vi "Module - Page Setup.vi"(11 "Stop":bool) -> ()   [LabVIEW 2020]
uses:
  Control/Setup - Sequence Data.ctl
  Control/Setup - Sequence Data Label.ctl
  Control/Setup - State.ctl
  Control/Data to Execute.ctl
  Control/Transaction Info.ctl
  Control/Product Info.ctl
  Control/Acceptance Criteria Info.ctl
  Control/Execution Info.ctl
  Control/Results Info.ctl
  Control/State - FGV.ctl
  Control/State - eFGV.ctl
  Control/Section.ctl
  <vilib>/Utility/NIReport.llb/Report Type.ctl
  7311f70c-db24-4098-937e-a840d3f1464f.vi
  babc2730-5d00-47f3-8067-32ba08f41054.vi
  b5994df8-9a62-4c2b-b0b7-1cda760cb50f.vi
  133289ce-597c-4077-9071-527faaeab83e.vi
  50162af0-f45e-4f35-a68f-88f28c3fa732.vi
  <vilib>/Utility/config.llb/Read Key (String).vi
  <vilib>/addons/_office/excel.llb/Excel Get Data ([str]).vi
  <vilib>/Comparison/Equal/Equal Functor/Equal Functor.lvclass
  <vilib>/Utility/NIReport.llb/NI_report.lvclass
  <vilib>/Utility/config.llb/NI_LVConfig.lvlib
  <vilib>/Utility/file.llb/Read Delimited Spreadsheet (string).vi
  <vilib>/Utility/NIReport.llb/NI_ReportGenerationCore.lvlib
  <vilib>/Utility/NIReport.llb/Excel/NI_Excel.lvclass
  <vilib>/addons/_office/NI_ReportGenerationToolkit.lvlib
panel:
  in  "Load Excel":bool
  in  "template (empty)":path
  in  "Tab Control":enum32{"Tests", "Misc."}(tab)=enum."Misc."
  in  "Btn.ClearRunSequence":bool caption="Run All"
  in  "Btn.RunSequence":bool caption="Run All"
  in  "ComboBox.SelectTestSequence":string(combo) caption="Test Sequence"
  in  "Remove Multi test":bool caption="Remove Sensor"
  in  "Add Multi test":bool caption="Add Sensor"
  in  "Header multi-test 3":T1={"Seq.SelectRun 4"="Select", "Seq.Done"="Status", "Seq.No"="Run?", "Seq.No 2"="Test Sequence", "Seq.No 3"="No.", "Seq.No 4"="Test Req. ID", "Seq.No 5"="Test Requirement", "Seq.No 6"="Variance", "Seq.No 7"="Test Procedure", "Seq.No 8"="Section", "Seq.No 9"="Test Bunker", "Seq.No 10"="Test Media", "Seq.No 11"="Test Pressure (psi)", "Seq.No 12"="Cycle", "Seq.No 13"="Holding time (hh:mm)", "Seq.No 14"="Chart Scale", "Seq.No 15"="Blowdown? (y/n)", "Seq.No 16"="Actuator Pressure (psi)", "Seq.No 17"="Max. Blowdown Pressure (psi)"}
  in  "MCListbox.Sequence List":T2[](array[typedef])
  in  "Enum.Permitted Hold Pressure Drop":enum16{"%", "psi"}(ring)
  in  "Enum.Max Start Hold Pressure":enum16{"%", "psi"}(ring)
  in  "Add Additional Ref Procedure":bool caption="Add Sensor"
  in  "Remove Additional Ref Procedure":bool caption="Remove Sensor"
  in  "Remove Sensor":bool
  in  "Add Tool":bool caption="Add Sensor"
  in  "Remove Tools":bool caption="Remove Sensor"
  in  "Add Sensor":bool
  in  "List.Tool":string(combo)
  in  "Header.Tool":T3={"Type "="Type", "Id"=" ID", "Description"="Description", "Serial No"="Serial No"} caption="Header Tool"
  in  "Label.Tools":string="Tools" caption="Tools"
  out "Output Set Description":string caption="Output Set Company"
  in  "ListBox.Output Set":string(combo)="1001.xltx" caption="Output Set"
  in  "Label.Result":string="Result" caption="Result"
  in  "List.Sensor":string(combo)
  in  "Label.Sensor":string="Sensor" caption="Sensor"
  out "Indicator.Sub Operation":string caption="Sub Operation"
  out "Indicator.Confirmation No":u32 caption="Confirmation No"
  out "Indicator.Operation":string caption="Operation"
  out "Indicator.Sequence No":u16 caption="Sequence No"
  in  "Label.Production Order Details":string="Production Order Details" caption="Production Order Details"
  out "Indicator.Order Number":u32 caption="Order Number"
  in  "Table.Procedure No./Ref.":i32(listbox)
  in  "Label.Execution":string="Execution" caption="Execution"
  in  "Label.Acceptance Criteria":string="Acceptance Criteria" caption="Acceptance Criteria"
  in  "Auto Stop Test":bool caption="Automatic Stop Test after Hold Time Countdown"
  in  "Auto Set Marker":bool=TRUE caption="Automatic set start marker upon pressure stabilized"
  in  "Permitted Hold Pressure Drop":dbl=3.0 caption="Permitted Holding Pressure Drop" min=0.0 max=100.0
  in  "Max Start Hold Pressure":dbl=3.0 caption="Maximum Start Of Holding Pressure" min=0.0 max=100.0
  in  "Listbox.PSL":string(combo) caption="PSL"
  in  "Listbox.Rev.":string(combo) caption="Rev."
  in  "Listbox.Additional Procedures No./Ref.":string(combo) caption="Additional Procedures No./Ref."
  in  "Label.Additional Procedures No./Ref.":string="Additional Procedures No./Ref." caption="Additional Procedures No./Ref."
  in  "Table.Sensor":i32(listbox) caption="Detail Sensor"
  in  "Header.Sensor":T4={"Type "="Type", "Id"=" ID", "Description"="Description", "Serial No"="Serial No", "LP"="LP"} caption="Header Detail Sensor"
  in  "Table.Tool":i32(listbox) caption="Detail Sensor"
  in  "Pressure Unit":string
  in  "List SN":i32(listbox)
  in  "Test System Description":string
  in  "Rework":bool caption="Rework?"
  in  "Ref Order No.":dbl caption="Ref. Order No."
  in  "NCR No.":string
  in  "Sales Order":u32
  in  "Procedure No./Ref.":string(combo) caption="Test Document No./Ref."
  in  "Save":bool
  in  "Edit":bool
  in  "Tab Control 2":T5(tab)
  in  "New":bool
  in  "Copy":bool
  in  "Remove SN":bool
  in  "Add SN":bool
  in  "Auto":bool
  in  "Notes":string
  in  "Input SN":string
  out "Working Pressure":string
  in  "Test Category":string
  in  "Test System":string(combo)
  in  "PSL":string
  in  "Rev.":string
  in  "Product Category":string(combo)
  in  "BOM Rev.":dbl
  in  "Material Description":string
  in  "Material":u32
  in  "Item No.":u32
  in  "Project":string
  in  "Customer Description":string
  in  "Customer":u32
  in  "Quantity":u16=1 min=1 step=1
  in  "Order Number":u32
  in  "Search":bool
  in  "Transaction Number":u32 caption="Transaction No."
  # "SETUP"
  # "PSL"
  # "Rev."
  # "on top of the test pressure"
  # "per hour (vs. start holding pressure)"
  # "Maximum Start of Holding Pressure"
  # "Pressure Holding Pressure Drop"
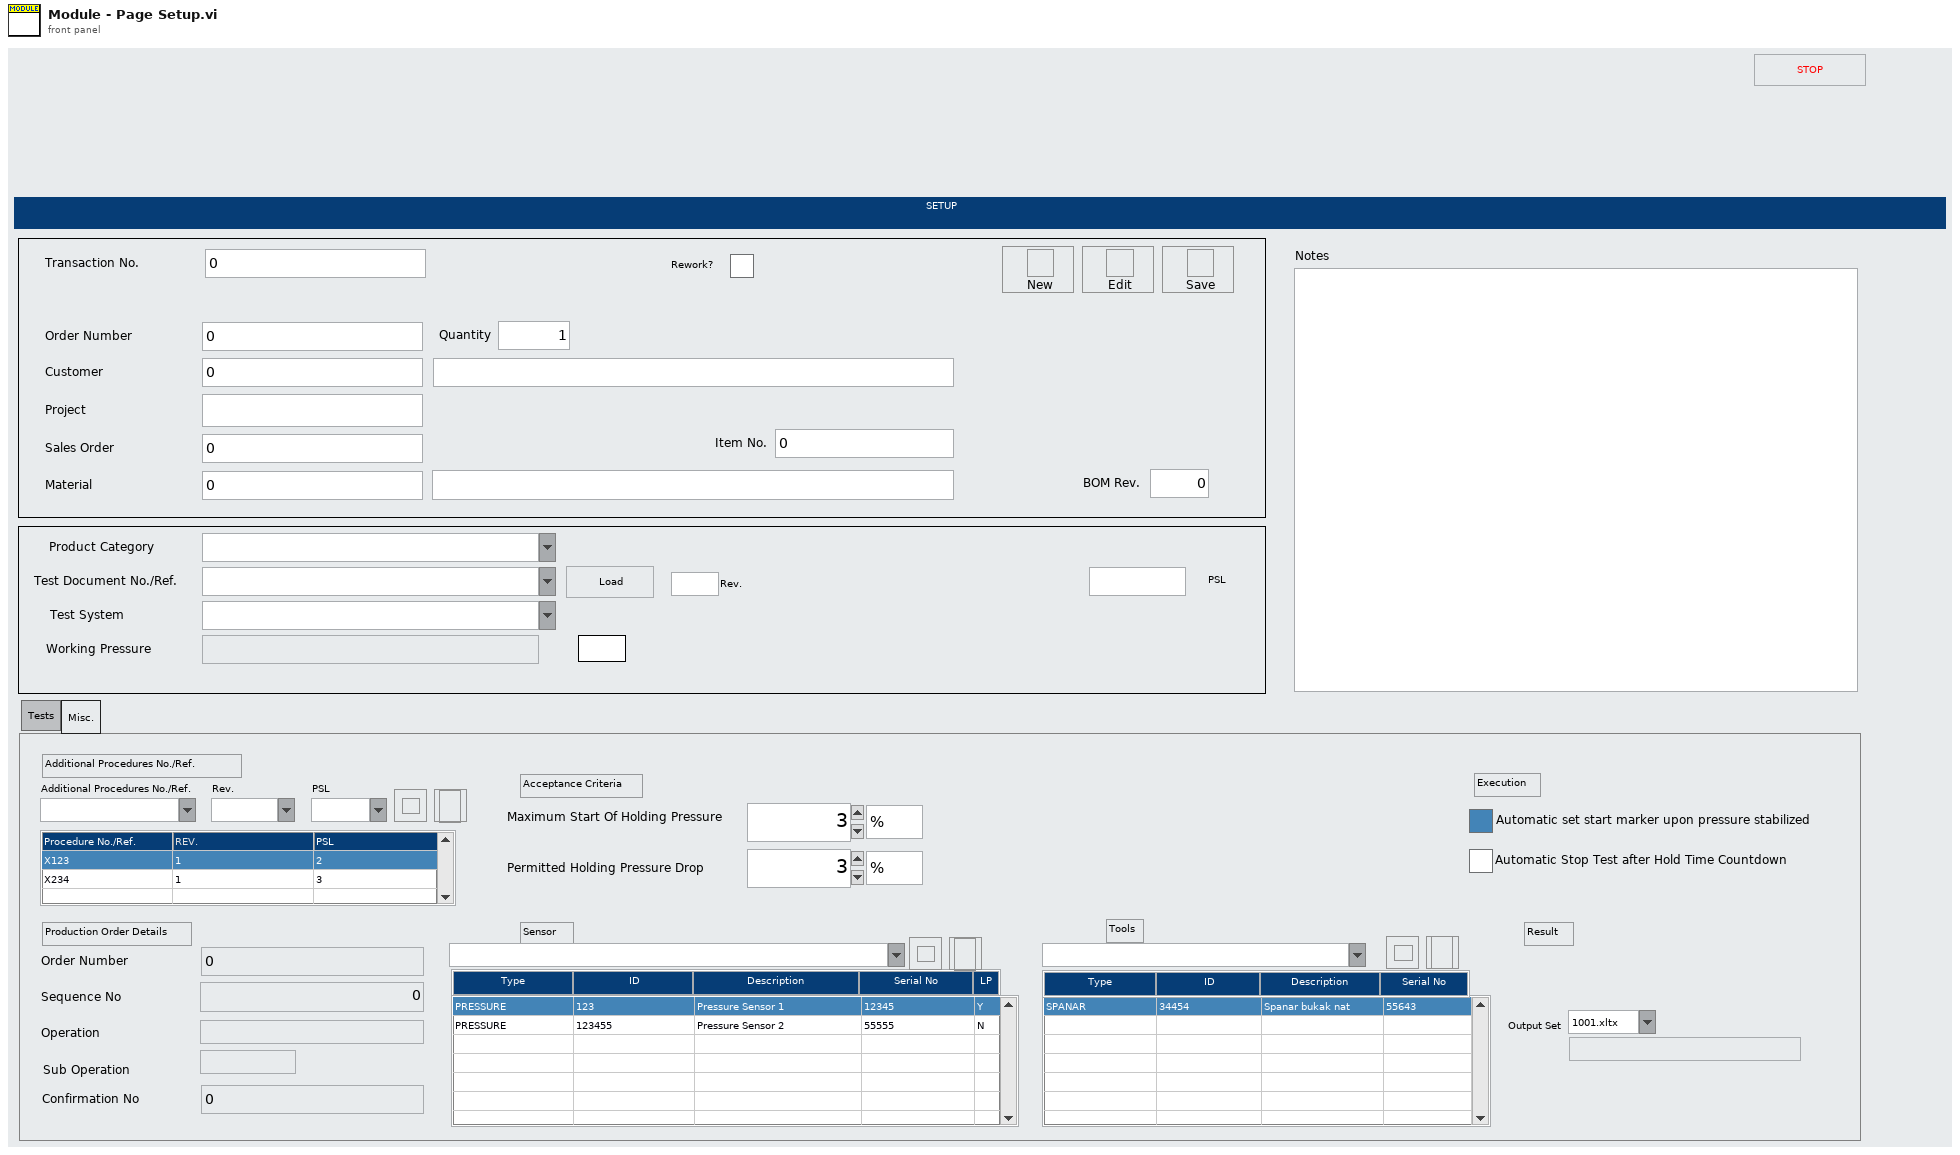
[diagram p1: front panel]
types:
  T1 = typedef "Setup - Sequence Data Label.ctl" = cluster{"Seq.SelectRun 4":string, "Seq.Done":string, "Seq.No":string, "Seq.No 2":string, "Seq.No 3":string, "Seq.No 4":string, "Seq.No 5":string, "Seq.No 6":string, "Seq.No 7":string, "Seq.No 8":string, "Seq.No 9":string, "Seq.No 10":string, "Seq.No 11":string, "Seq.No 12":string, "Seq.No 13":string, "Seq.No 14":string, "Seq.No 15":string, "Seq.No 16":string, "Seq.No 17":string}
  T2 = typedef "Setup - Sequence Data.ctl" = cluster{"Seq.Select":bool, "Seq.Status":u32, "Seq.Run":bool, "Seq.TestSequence":string, "Seq.No":string, "Seq.ReqID":string, "Seq.TestReq":string, "Seq.Variance":string, "Seq.TestProcedure":string, "Seq.Section":string, "Seq.TestBunker":string, "Seq.TestMedia":string, "Seq.TestPressure":string, "Seq.Cycle":string, "Seq.HoldingTime":string, "Seq.ChartScale":string, "Seq.BDIndicator":string, "Seq.ActuatorPressure":string, "Seq.MaxBDPressure":string}
  T3 = cluster{"Type ":string, "Id":string, "Description":string, "Serial No":string}
  T4 = cluster{"Type ":string, "Id":string, "Description":string, "Serial No":string, "LP":string}
  T5 = enum32{"Others                ", "Multi-tests       "}
  T6 = typedef "Data to Execute.ctl" = cluster{"Transaction Info":T7, "Product Info":T8, "Misc - Additional Refs":string[][], "Misc - Sensors":string[][], "Misc - Tools":string[][], "Acceptance Criteria Info":T9, "Execution Info":T10, "Results Info":T11, "Notes":string}
  T7 = typedef "Transaction Info.ctl" = cluster{"Transaction Number":u32, "Order Number":u32, "Quantity":u16, "Customer":u32, "Customer Description":string, "Project":string, "Sales Order":u32, "Material":u32, "Material Description":string, "Rework":bool, "NCR No.":string, "Ref Order No.":dbl, "Item No.":u32, "BOM Rev.":dbl}
  T8 = typedef "Product Info.ctl" = cluster{"Product Category":string, "Procedure No./Ref.":string, "Test System":string, "Test System Description":string, "Working Pressure":string, "Pressure Unit":string, "Rev.":string, "PSL":string}
  T9 = typedef "Acceptance Criteria Info.ctl" = cluster{"Max Start Hold Pressure":dbl, "Enum.Max Start Hold Pressure":enum16{"%", "psi"}, "Permitted Hold Pressure Drop":dbl, "Enum.Permitted Hold Pressure Drop":enum16{"%", "psi"}}
  T10 = typedef "Execution Info.ctl" = cluster{"Auto Set Marker":bool, "Auto Stop Test":bool}
  T11 = typedef "Results Info.ctl" = cluster{"ListBox.Output Set":string, "Output Set Description":string}
  T12 = cluster{"T_Out":i32, "Event Ref":refnum<event-registration>, "Product Category":string, "Seq.AllList":T2[], "Seq.ShownList":T2[], "Seq.HiddenList":T2[], "Procedure No.":string, "File String":string[], "Data to Execute":T6}
  T13 = typedef "Setup - State.ctl" = enum16{"Init", "Register Event", "Read Config File", "Get Output Set List", "Idle", "Get product info", "Read sequence csv", "Get Sequence List", "Get Transaction Info", "Get product Info", "Get Misc - Additional Refs", "Get Misc - Sensors", "Get Misc - Tools", "Get Misc - Accept Criteria", "Get Misc - Execution", "Get Misc - Results", "Get Misc - Notes", "Check Folder Exist", "Create Folder", "Send to Execute", "Close"}
  T14 = typedef "State - FGV.ctl" = enum16{"Write", "Read"}
  T15 = typedef "State - eFGV.ctl" = enum16{"Init", "Read", "Write", "Exit"}
  T16 = typedef "Section.ctl" = enum16{"Software Setup", "Config", "Setup", "Network Stream", "MQTT Client", "Setting", "Sample Interval", "Calibration", "Pre-Ranging", "Overrun", "Static", "Filter", "Properties", "Alarm", "Device", "Logging"}
  T17 = enum8{"Enabled", "Disabled", "Disabled and Grayed Out"}
  T18 = enum16{"maximized", "minimized", "normal", "no change"}
  T19 = typedef "NI_ReportGenerationCore.lvlib/Report Type.ctl" = enum16{"HTML", "Word", "Excel"}
  T20 = typedef "NI_LVConfig.lvlib/Config Data RefNum.ctl" = refnum<k1>
  T21 = cluster{"Type":string, "ID":string, "Description":string, "Serial No.":string, "Low Pressure?":bool}
  T22 = cluster{"Type":string, "ID":string, "Description":string, "Serial No.":string}
  T23 = cluster{"Transaction Number":u32, "Order Number":u32, "Quantity":u16, "Customer":u32, "Customer Description":string, "Project":string, "Sales Order":u32, "Material":u32, "Material Description":string, "Rework":bool, "NCR No.":string, "Ref Order No.":dbl, "Item No.":u32, "BOM Rev.":dbl}
  T24 = cluster{"Product Category":string, "Procedure No./Ref.":string, "Test System":string, "Test System Description":string, "Working Pressure":string, "Pressure Unit":string, "Rev.":string, "PSL":string}
  T25 = cluster{"Max Start Hold Pressure":dbl, "Enum.Max Start Hold Pressure":enum16{"%", "psi"}, "Permitted Hold Pressure Drop":dbl, "Enum.Permitted Hold Pressure Drop":enum16{"%", "psi"}}
  T26 = cluster{"Auto Set Marker":bool, "Auto Stop Test":bool}
  T27 = cluster{"ListBox.Output Set":string, "Output Set Description":string}
  T28 = enum32{"invalid app kind", "Development System", "Run Time System", "Student Edition", "Embedded LabVIEW", "Evaluation", "Custom"}
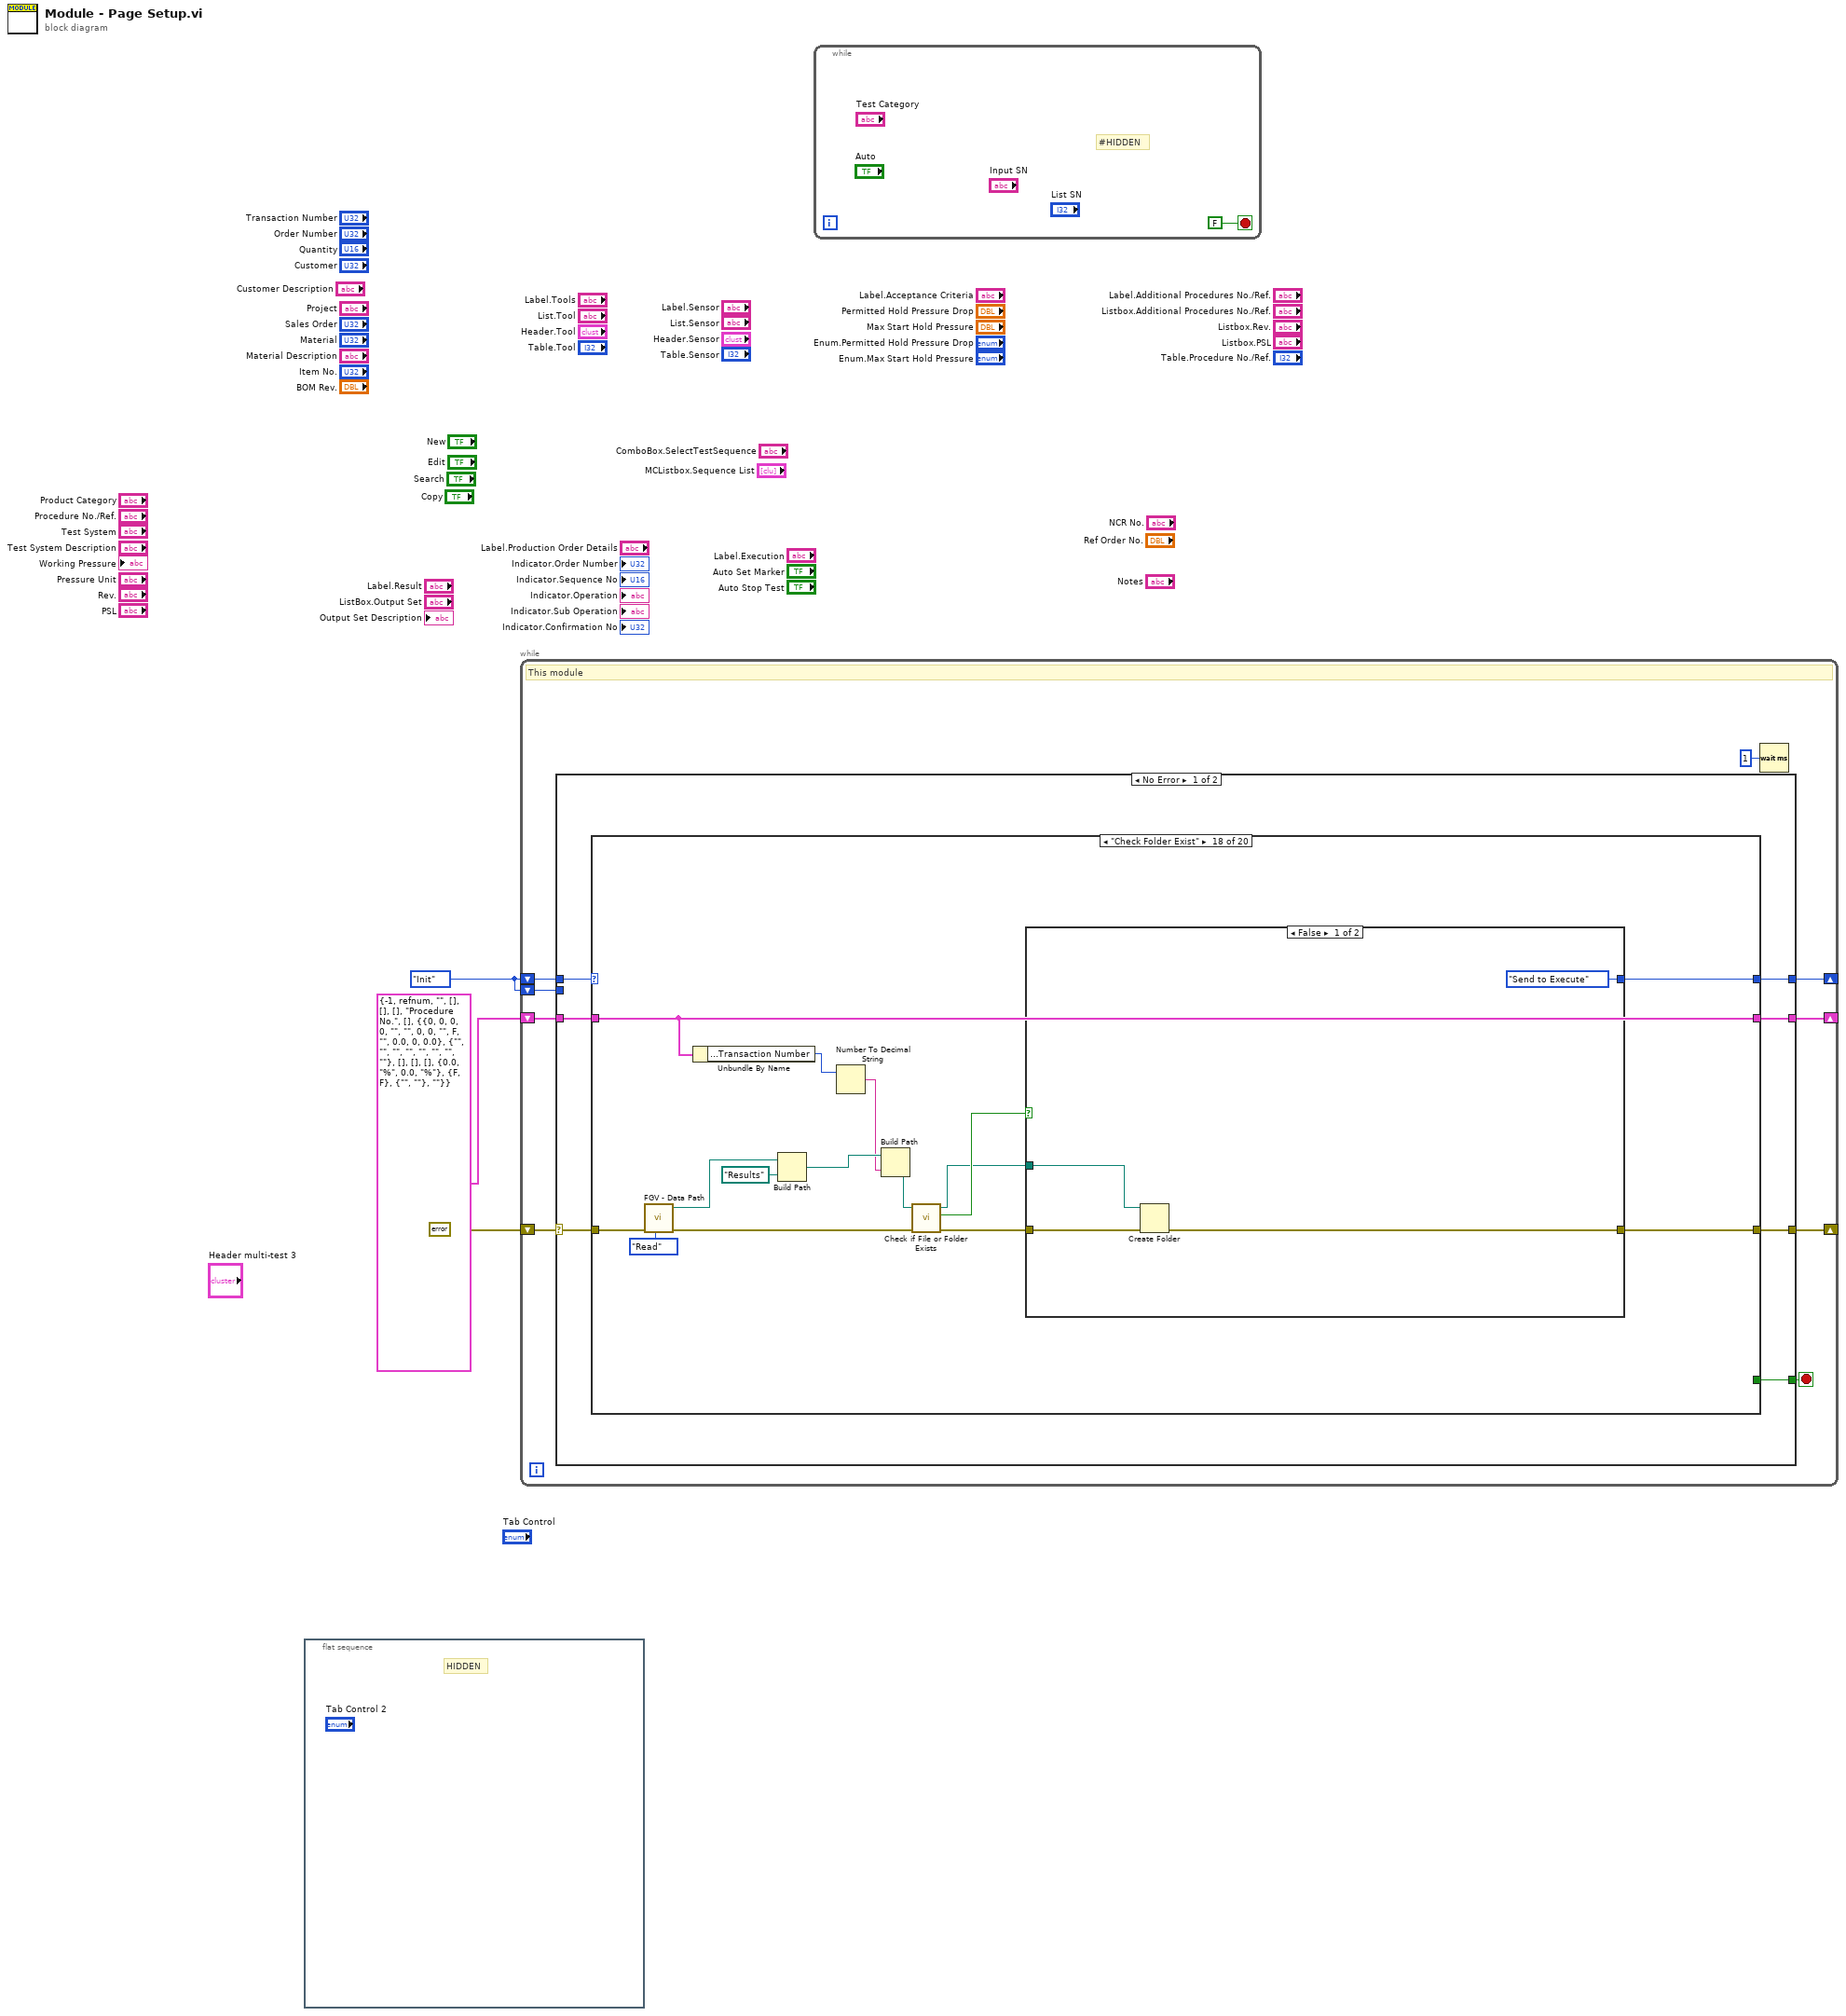
[diagram p0: block diagram]
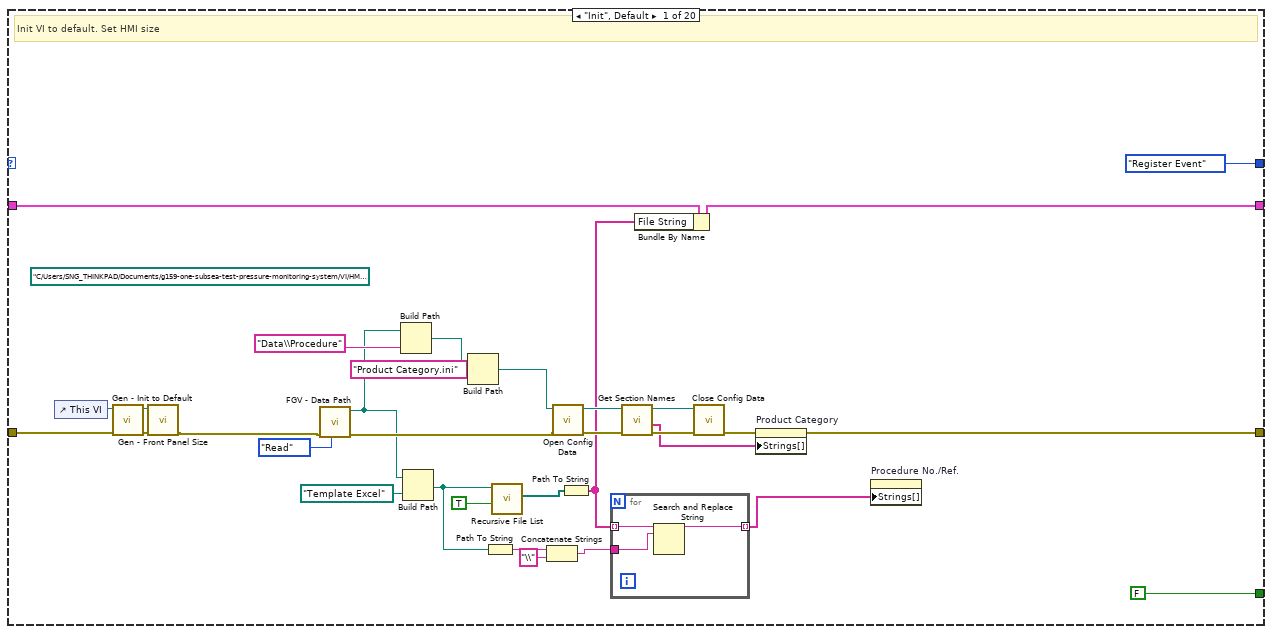
[diagram p2: hidden frame]
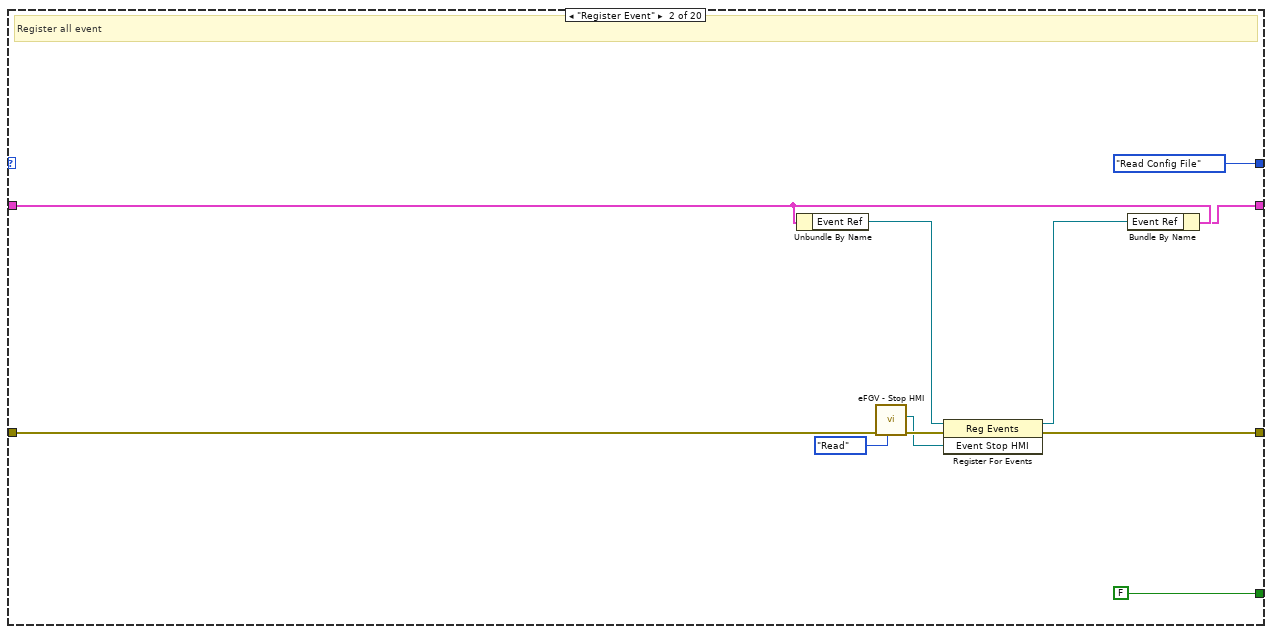
[diagram p3: hidden frame]
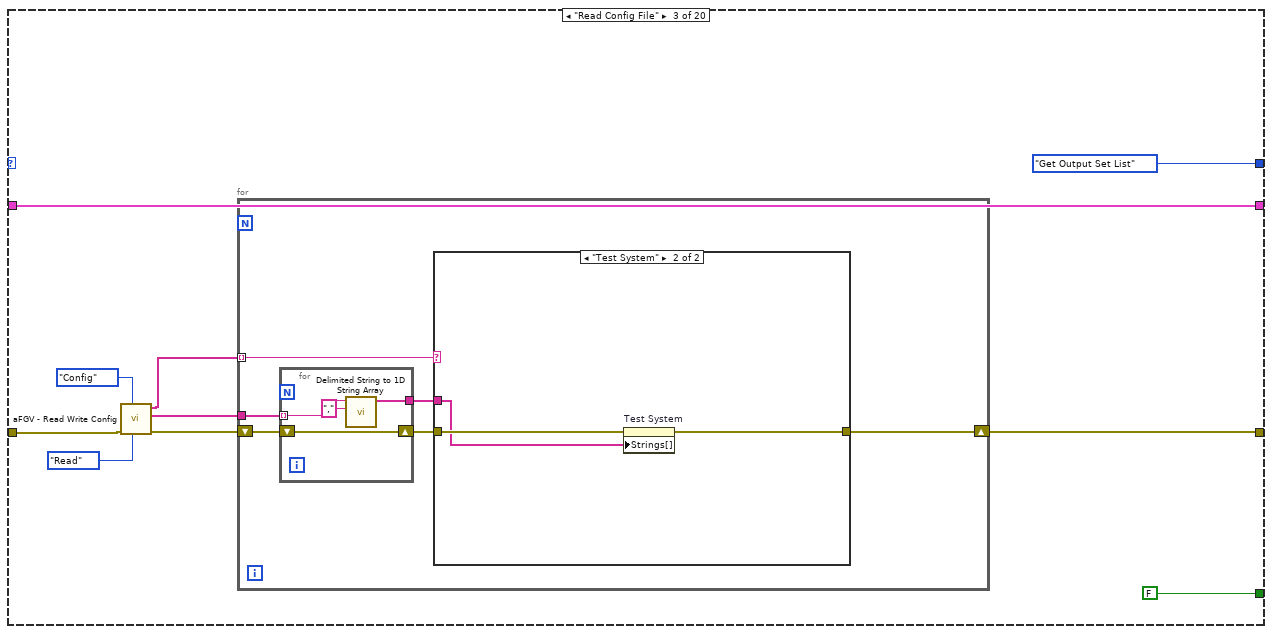
[diagram p4: hidden frame]
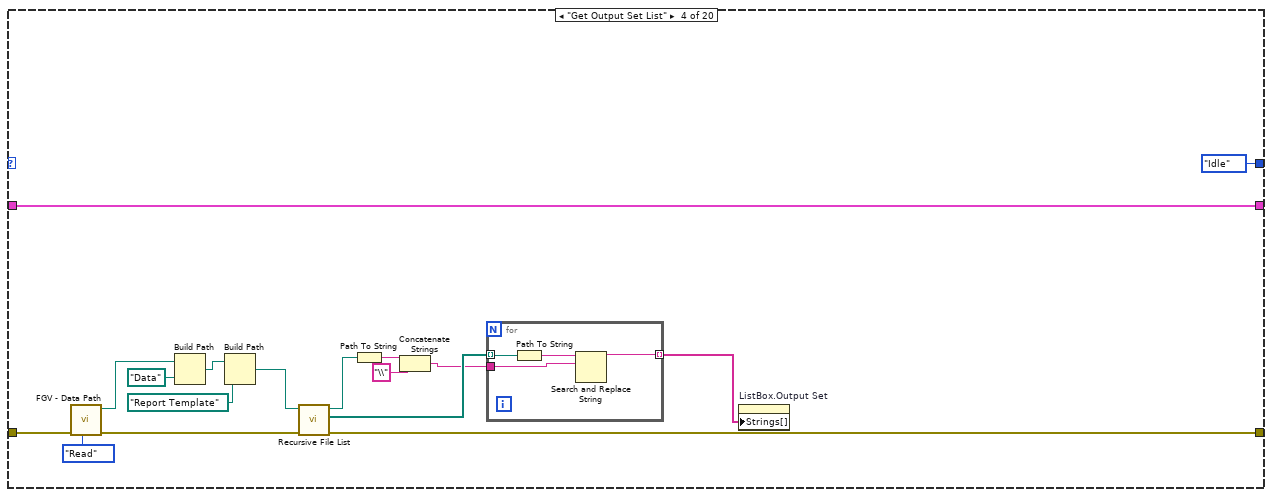
[diagram p6: hidden frame]
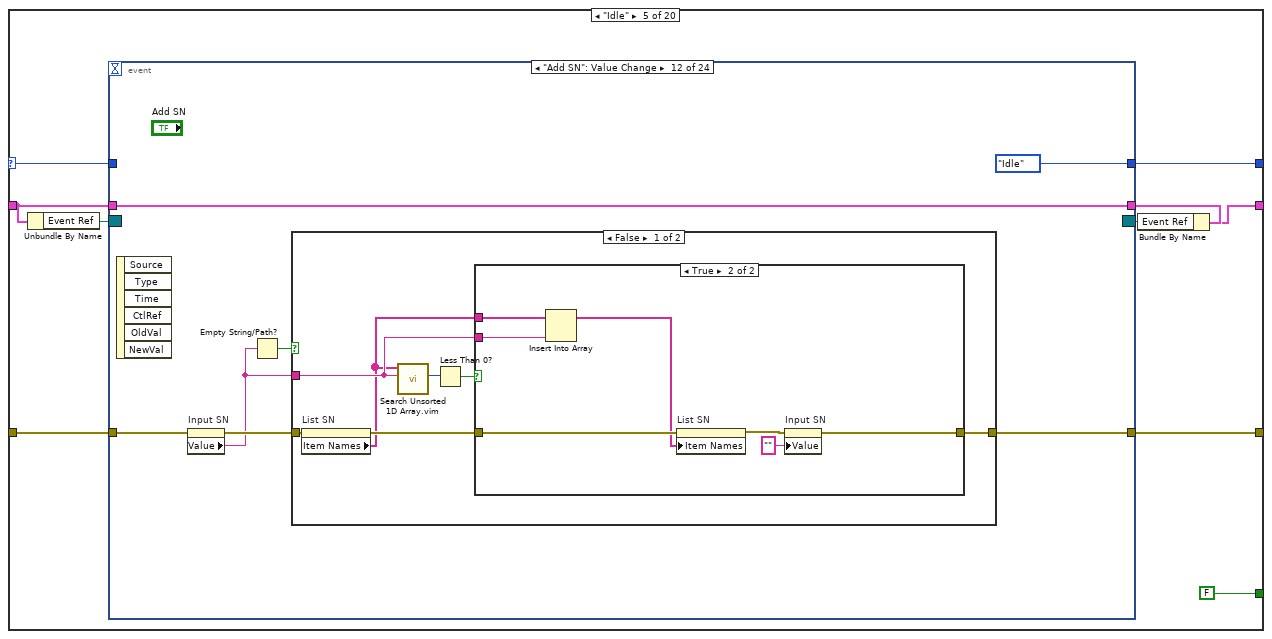
[diagram p7: hidden frame]
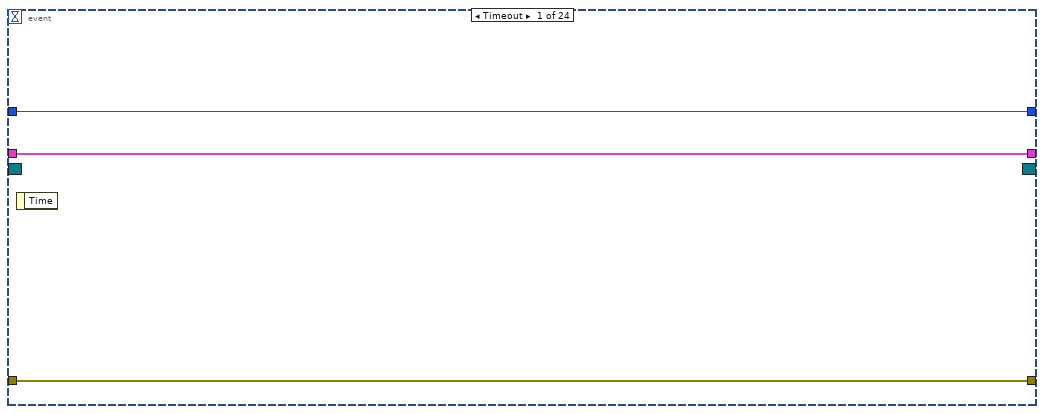
[diagram p8: hidden frame]
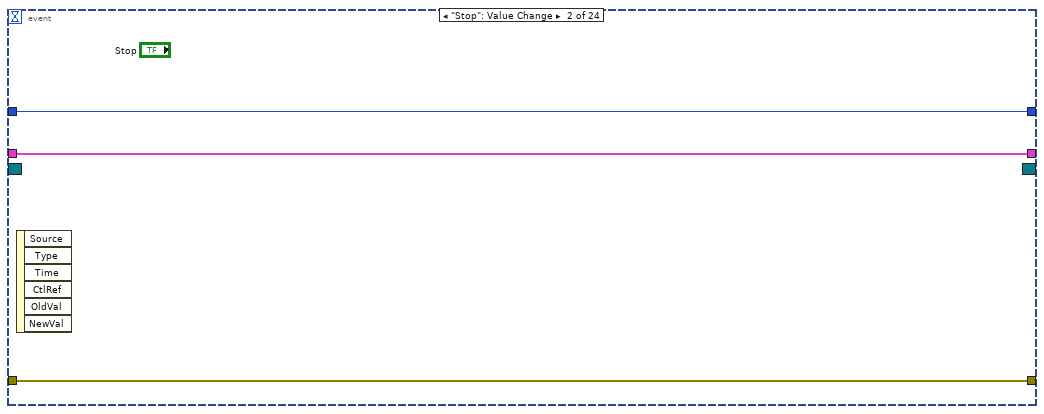
[diagram p9: hidden frame]
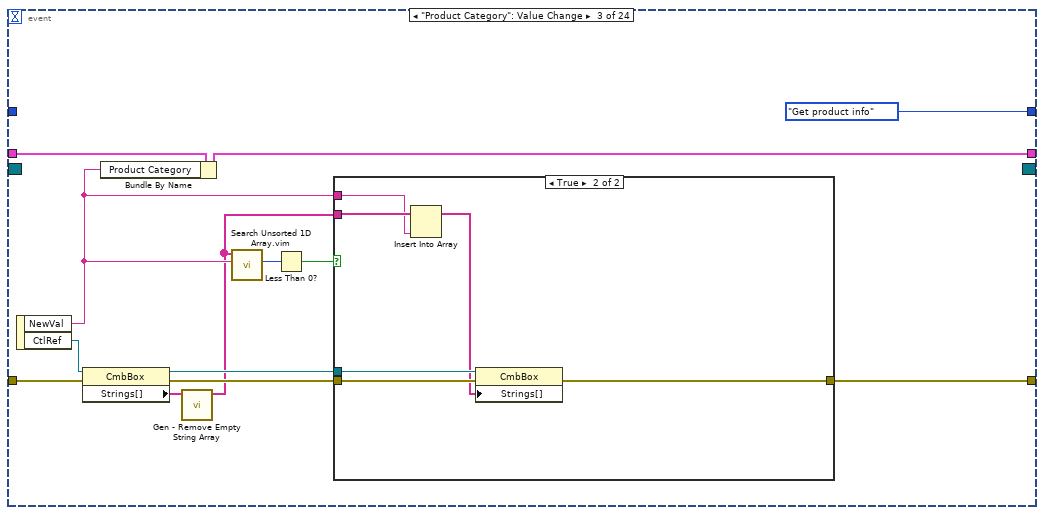
[diagram p10: hidden frame]
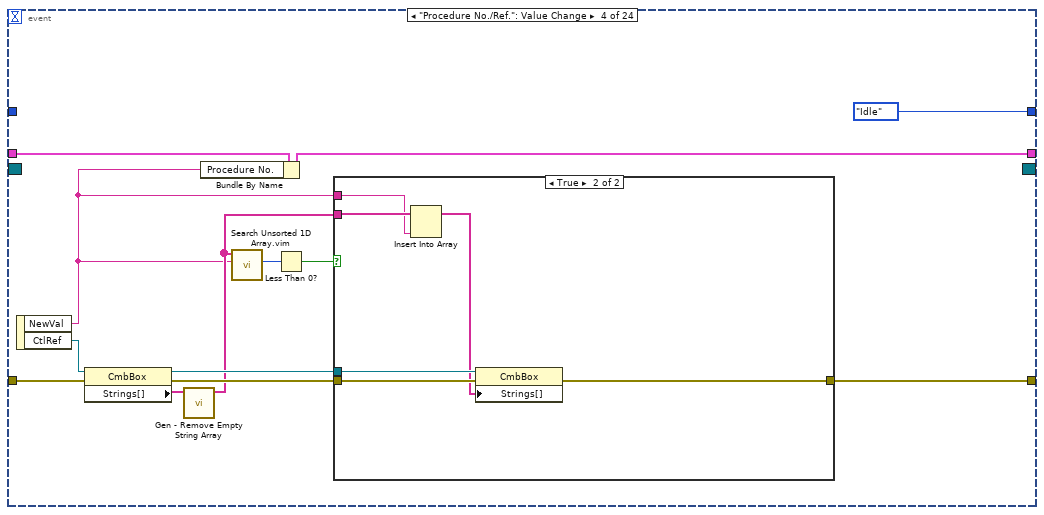
[diagram p12: hidden frame]
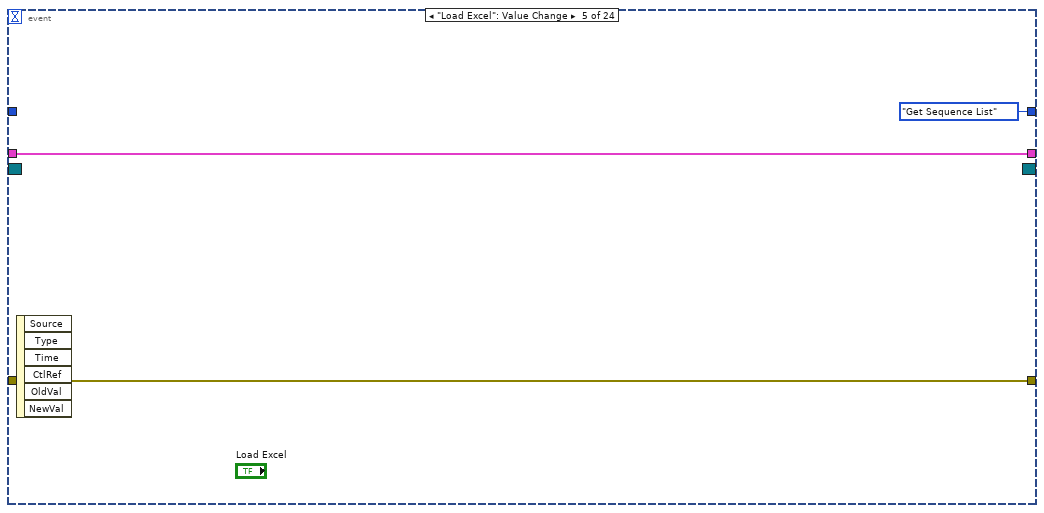
[diagram p14: hidden frame]
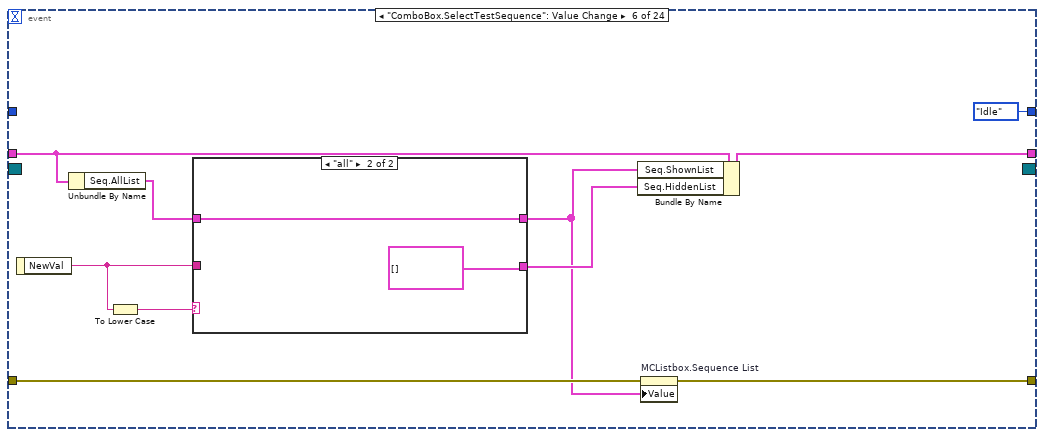
[diagram p15: hidden frame]
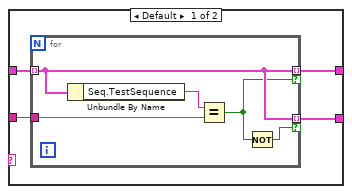
[diagram p16: hidden frame]
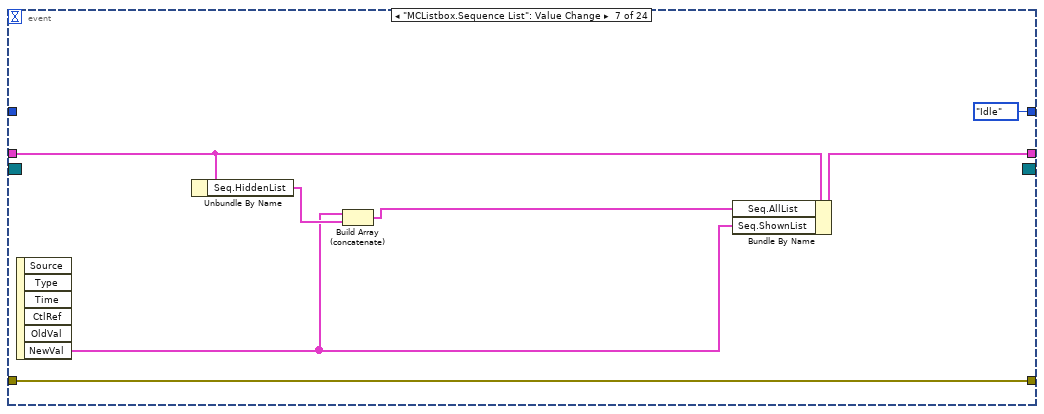
[diagram p17: hidden frame]
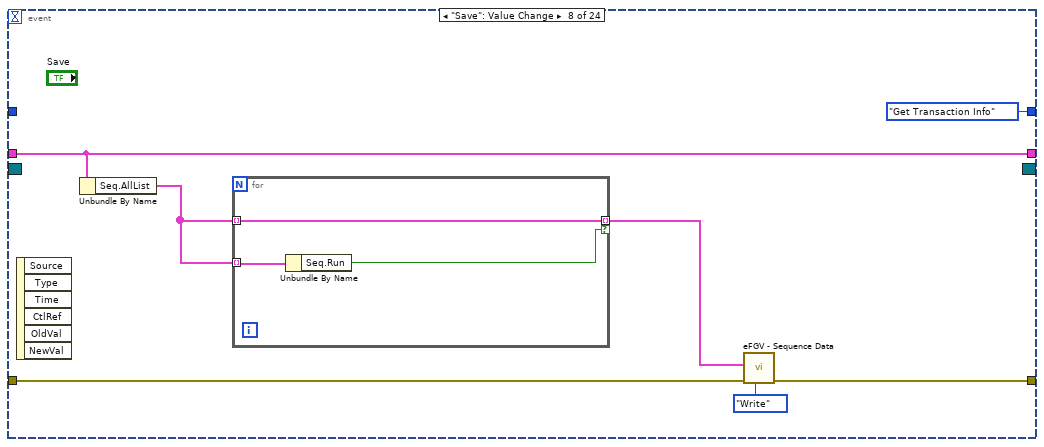
[diagram p18: hidden frame]
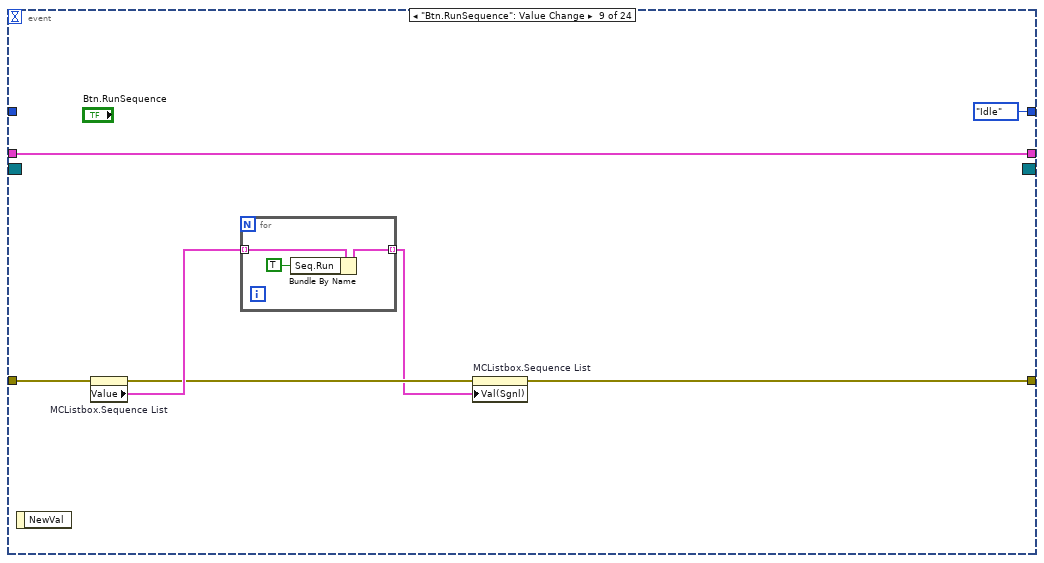
[diagram p19: hidden frame]
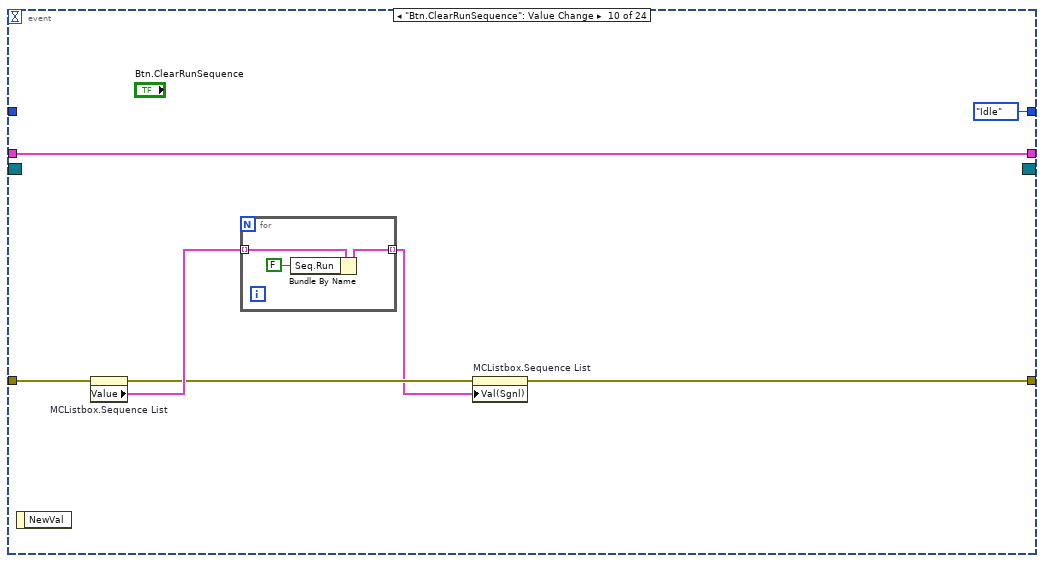
[diagram p20: hidden frame]
diagram:
  w1 = Setup_-_State."Init"
  n1 = flat-sequence {
    frame #0 {
      # "HIDDEN"
    }
  }
  n2 = while {
    shift-right: [w8] -> _
    shift-left: w1 -> [w10]
    shift-right: [w11] -> _
    shift-left: errorcluster {"status"=FALSE, "code"=0, "source"=""} ("Error In") -> [w12]
    shift-right: [w6] -> _
    shift-left: T12 {"T_Out"=-1, "Event Ref"=refnum, "Product Category"="", "Seq.AllList"=[], "Seq.ShownList"=[], "Seq.HiddenList"=[], "Procedure No."="Procedure No.", "File String"=[], "Data to Execute"={"Transaction Info"={"Transaction Number"=0, "Order Number"=0, "Quantity"=0, "Customer"=0, "Customer Description"="", "Project"="", "Sales Order"=0, "Material"=0, "Material Description"="", "Rework"=FALSE, "NCR No."="", "Ref Order No."=0.0, "Item No."=0, "BOM Rev."=0.0}, "Product Info"={"Product Category"="", "Procedure No./Ref."="", "Test System"="", "Test System Description"="", "Working Pressure"="", "Pressure Unit"="", "Rev."="", "PSL"=""}, "Misc - Additional Refs"=[], "Misc - Sensors"=[], "Misc - Tools"=[], "Acceptance Criteria Info"={"Max Start Hold Pressure"=0.0, "Enum.Max Start Hold Pressure"=enum."%", "Permitted Hold Pressure Drop"=0.0, "Enum.Permitted Hold Pressure Drop"=enum."%"}, "Execution Info"={"Auto Set Marker"=FALSE, "Auto Stop Test"=FALSE}, "Results Info"={"ListBox.Output Set"="", "Output Set Description"=""}, "Notes"=""}} -> [w7]
    shift-left: w1 -> [w4]
    stop <- w9 stop-if-true
    # "This module"
    n3 = case shown="No Error" w12 {
      selector: w12 -> [w18 w633]
      tunnel: w10 -> [w17 w638]
      tunnel: [w19 w634] -> w11
      tunnel: [w16 FALSE] -> w9
      tunnel: [w15 w638] -> w8
      tunnel: w7 -> [w14 w637]
      tunnel: [w13 w637] -> w6
      tunnel: w4 -> [_ w630]
      frame No Error {
        n4 = case shown="\"Check Folder Exist\"" w17 {
          selector: w17 -> [_ _ _ _ w115 _ _ _ _ _ _ _ _ _ _ _ _ _ _ w627]
          tunnel: [w39 w65 w68 w98 w120 w433 w462 w488 w534 w547 w551 w557 w563 w574 w581 w588 w593 w596 w622 w628] -> w19
          tunnel: w18 -> [w51 w63 w73 w104 w119 w434 w461 w489 w534 w547 w552 w558 w564 w574 w581 w588 w593 w608 w623 w629]
          tunnel: [FALSE FALSE FALSE _ FALSE FALSE FALSE _ FALSE _ _ _ _ _ _ _ _ _ _ TRUE] -> w16
          tunnel: [Setup_-_State."Register Event" Setup_-_State."Read Config File" Setup_-_State."Get Output Set List" Setup_-_State."Idle" w117 Setup_-_State."Read sequence csv" Setup_-_State."Idle" Setup_-_State."Idle" Setup_-_State."Get product Info" Setup_-_State."Get Misc - Additional Refs" Setup_-_State."Get Misc - Sensors" Setup_-_State."Get Misc - Tools" Setup_-_State."Get Misc - Accept Criteria" Setup_-_State."Get Misc - Execution" Setup_-_State."Get Misc - Results" Setup_-_State."Get Misc - Notes" Setup_-_State."Check Folder Exist" w597 Setup_-_State."Idle" w627] -> w15
          tunnel: w14 -> [w49 w59 w75 w106 w114 w432 w465 w485 w532 w546 w553 w559 w565 w573 w580 w587 w592 w605 w620 w625]
          tunnel: [w22 w57 w75 w106 w112 w432 w465 w487 w530 w537 w550 w556 w562 w568 w577 w584 w591 w605 w620 w625] -> w13
          frame "Init", Default {
            (unwired) path "C:/Users/SNG_THINKPAD/Documents/g159-one-subsea-test-pressure-monitoring-system/VI/HMI/Data/Data/Procedure/Product Category.ini" ("configuration file path")
            # "Init VI to default. Set HMI size"
            n5 = control-ref of="This VI"() -> (w47:refnum<vi>)
            n6 = call "Gen - Init to Default.vi"("Error in"=w51, "This VI"=w47) -> ("Error out"=w50:errorcluster, "This VI Copy"=w46:refnum<vi>)  [unwired: 8 in]
            n7 = call "Gen - Front Panel Size.vi"("Error In"=w50, "This VI"=w46) -> ("Error Out"=w36:errorcluster)  [unwired: 9 in]
            n8 = call "FGV - Data Path.vi"("FGV State"=State_-_FGV."Read", "Error In"=w36) -> ("Error Out"=w35:errorcluster, "Path Out"=w31:path)  [unwired: 8 in]
            n9 = Build Path(base path=w31, name or relative path="Data\\Procedure") -> (appended path=w34:path)
            n10 = Build Path(base path=w31, name or relative path=path "Template Excel") -> (appended path=w27:path)
            n11 = Build Path(base path=w34, name or relative path="Product Category.ini") -> (appended path=w32:path)
            n12 = Path To String(path=w27) -> (string=w25:string)
            n13 = call <vilib>:"Recursive File List.vi"("Continue Recursing on Error? (F)"=TRUE, "Folder Path"=w27) -> ("All Files in Dir"=w28:path[])  [unwired: 5 in, 4 out]
            n14 = Concatenate Strings(w25, "\\" ("string")) -> (w23:string)
            n15 = call <vilib>:"Open Config Data.vi"("error in (no error)"=w35, "configuration file path"=w32) -> ("error out"=w45:errorcluster, "refnum"=w42:T20)  [unwired: 7 in, 1 out]
            n16 = Path To String(path=w28) -> (string=w21:string[])
            n17 = for {
              tunnel: w21 -> [w54] mode=indexing
              tunnel: w23 -> [w53]
              tunnel: [w52] -> w26 mode=indexing
              n18 = Search and Replace String(input string=w54, search string=w53) -> (result string=w52:string)  [unwired: 6 in, 3 out]
            }
            n19 = call <vilib>:"Get Section Names.vi"("error in (no error)"=w45, "refnum"=w42) -> ("error out"=w43:errorcluster, "section names"=w40:string[], "refnum out"=w44:T20)  [unwired: 7 in]
            n20 = Bundle By Name(cluster=w49, "File String"=w21) -> (w22:T12)
            n21 = call <vilib>:"Close Config Data.vi"("error in (no error)"=w43, "refnum"=w44) -> ("error out"=w41:errorcluster)  [unwired: 8 in, 1 out]
            n22 = property on="Product Category" class="CmbBox"(error in=w41, "Strings[]"=w40) -> (error out=w39:errorcluster)  [unwired: 1 in, 1 out]
            n23 = property on="Procedure No./Ref." class="CmbBox"("Strings[]"=w26) -> ()  [unwired: 2 in, 2 out]
          }
          frame "Register Event" {
            # "Register all event"
            n24 = Unbundle By Name(w59) -> ("Event Ref"=w58:refnum<event-registration>)
            n25 = call "eFGV - Stop HMI.vi"("Action"=State_-_eFGV."Read", "Error In"=w63) -> ("Error Out"=w64:errorcluster, "Event Stop HMI"=w61:refnum<user-event>)  [unwired: 7 in, 1 out]
            n26 = register-events(reference=w58, error in=w64, w61) -> (reference out=w56:refnum<event-registration>, error out=w65:errorcluster)
            n27 = Bundle By Name(cluster=w59, "Event Ref"=w56) -> (w57:T12)
          }
          frame "Read Config File" {
            n28 = call "aFGV - Read Write Config.vi"("State"=enum16{"Read", "Write", "Delete"}."Read", "Section"=Section."Config", "Error In"=w73) -> ("Error Out"=w69:errorcluster, "Data out"=w66:string[], "Key Names"=w67:string[])  [unwired: 6 in]
            n29 = for {
              shift-right: [w81] -> w68
              shift-left: w69 -> [w79]
              tunnel: w67 -> [w80] mode=indexing
              tunnel: w66 -> [w77]
              n30 = for {
                shift-right: [w85] -> w78
                shift-left: w79 -> [w85]
                tunnel: w77 -> [w84] mode=indexing
                tunnel: [w82] -> w76
                n31 = call <vilib>:"Delimited String to 1D String Array.vi"("delimiter"=",", "delimited string"=w84) -> ("string array"=w82:string[])  [unwired: 9 in]
              }
              n32 = case shown="\"Test System\"" w80 {
                tunnel: w78 -> [w86 w89]
                tunnel: [w86 w88] -> w81
                tunnel: w76 -> [_ w87]
                frame Default {
                }
                frame "Test System" {
                  n33 = property on="Test System" class="CmbBox"(error in=w89, "Strings[]"=w87) -> (error out=w88:errorcluster)  [unwired: 1 in, 1 out]
                }
              }
            }
          }
          frame "Get Output Set List" {
            n34 = call "FGV - Data Path.vi"("FGV State"=State_-_FGV."Read", "Error In"=w104) -> ("Error Out"=w99:errorcluster, "Path Out"=w103:path)  [unwired: 8 in]
            n35 = Build Path(base path=w103, name or relative path=path "Data") -> (appended path=w101:path)
            n36 = Build Path(base path=w101, name or relative path=path "Report Template") -> (appended path=w97:path)
            n37 = call <vilib>:"Recursive File List.vi"("error in (no error)"=w99, "Folder Path"=w97) -> ("error out"=w98:errorcluster, "All Files in Dir"=w96:path[], "dup Folder Path"=w95:path)  [unwired: 5 in, 2 out]
            n38 = Path To String(path=w95) -> (string=w94:string)
            n39 = Concatenate Strings(w94, "\\" ("string")) -> (w92:string)
            n40 = for {
              tunnel: w96 -> [w110] mode=indexing
              tunnel: w92 -> [w108]
              tunnel: [w107] -> w91 mode=indexing
              n41 = Path To String(path=w110) -> (string=w109:string)
              n42 = Search and Replace String(input string=w109, search string=w108) -> (result string=w107:string)  [unwired: 6 in, 3 out]
            }
            n43 = property on="ListBox.Output Set" class="CmbBox"("Strings[]"=w91) -> ()  [unwired: 2 in, 2 out]
          }
          frame "Idle" {
            n44 = Unbundle By Name(w114) -> ("Event Ref"=w113:refnum<event-registration>)
            n45 = event shown="[11] \"Add SN\": Value Change" {
              selector: w113 -> [_ _ _ _ _ _ _ _ _ _ _ _ _ _ _ _ _ _ _ _ _ _ _ _]
              dyn-events: [_ _ _ _ _ _ _ _ _ _ _ _ _ _ _ _ _ _ _ _ _ _ _ _] -> w111
              timeout: _ -> [_ _ _ _ _ _ _ _ _ _ _ _ _ _ _ _ _ _ _ _ _ _ _ _]
              tunnel: [w123 w126 w129 w151 w169 w174 w197 w201 w210 w220 w230 w248 w273 w282 w305 w314 w337 w353 w363 w373 w388 w406 w411 w422] -> w120
              tunnel: w119 -> [w123 w126 w135 w156 w169 w175 w197 w202 w213 w223 w236 w252 w279 w289 w307 w316 w338 w360 w370 w380 w389 w406 w412 w423]
              tunnel: [w121 w124 Setup_-_State."Get product info" Setup_-_State."Idle" Setup_-_State."Get Sequence List" Setup_-_State."Idle" Setup_-_State."Idle" Setup_-_State."Get Transaction Info" Setup_-_State."Idle" Setup_-_State."Idle" Setup_-_State."Idle" Setup_-_State."Idle" Setup_-_State."Idle" Setup_-_State."Idle" Setup_-_State."Idle" Setup_-_State."Idle" Setup_-_State."Idle" Setup_-_State."Idle" Setup_-_State."Idle" Setup_-_State."Idle" Setup_-_State."Idle" Setup_-_State."Close" Setup_-_State."Idle" Setup_-_State."Idle"] -> w117
              tunnel: [w122 w125 w137 w148 w168 w177 w195 w204 w214 w224 w239 w253 w280 w290 w308 w318 w340 w362 w372 w382 w394 w405 w413 w424] -> w116
              tunnel: w114 -> [w122 w125 w139 w159 w168 w179 w194 w204 w214 w224 w239 w253 w280 w290 w308 w318 w340 w362 w372 w382 w394 w405 w413 w424]
              tunnel: w115 -> [w121 w124 _ _ _ _ _ _ _ _ _ _ _ _ _ _ _ _ _ _ _ _ _ _]
              event Timeout {
                n46 = event-data() -> ()  [unwired: 1 in, 1 out]
              }
              event "Stop": Value Change {
                n47 = event-data() -> ()  [unwired: 1 in, 6 out]
              }
              event "Product Category": Value Change {
                n48 = event-data() -> ("NewVal"=w132:string, "CtlRef"=w136:refnum<vi>)  [unwired: 1 in]
                n49 = property class="CmbBox"(reference=w136, error in=w135) -> (reference out=w130:refnum<vi>, error out=w131:errorcluster, "Strings[]"=w128:string[])
                n50 = Bundle By Name(cluster=w139, "Product Category"=w132) -> (w137:T12)
                n51 = call "Gen - Remove Empty String Array.vi"("Data Array"=w128) -> ("Data Out"=w127:string[])  [unwired: 10 in]
                n52 = call "Search Unsorted 1D Array.vim"("element"=w132, "unsorted 1D array"=w127) -> ("index of element"=w134:i32)  [unwired: 9 in]
                n53 = Less Than 0?(x=w134) -> (x < 0?=w133:bool)
                n54 = case shown="True" w133 {
                  tunnel: w127 -> [_ w146]
                  tunnel: w132 -> [_ w145]
                  tunnel: w131 -> [w140 w144]
                  tunnel: w130 -> [_ w143]
                  tunnel: [w140 w141] -> w129
                  frame False {
                  }
                  frame True {
                    n55 = Insert Into Array(array=w146, new element=w145) -> (w142:string[])  [unwired: 1 in]
                    n56 = property class="CmbBox"(reference=w143, error in=w144, "Strings[]"=w142) -> (error out=w141:errorcluster)  [unwired: 1 out]
                  }
                }
              }
              event "Procedure No./Ref.": Value Change {
                n57 = event-data() -> ("NewVal"=w147:string, "CtlRef"=w157:refnum<vi>)  [unwired: 1 in]
                n58 = property class="CmbBox"(reference=w157, error in=w156) -> (reference out=w152:refnum<vi>, error out=w153:errorcluster, "Strings[]"=w150:string[])
                n59 = call "Gen - Remove Empty String Array.vi"("Data Array"=w150) -> ("Data Out"=w149:string[])  [unwired: 10 in]
                n60 = Bundle By Name(cluster=w159, "Procedure No."=w147) -> (w148:T12)
                n61 = call "Search Unsorted 1D Array.vim"("element"=w147, "unsorted 1D array"=w149) -> ("index of element"=w155:i32)  [unwired: 9 in]
                n62 = Less Than 0?(x=w155) -> (x < 0?=w154:bool)
                n63 = case shown="True" w154 {
                  tunnel: w149 -> [_ w166]
                  tunnel: w147 -> [_ w165]
                  tunnel: w153 -> [w160 w164]
                  tunnel: w152 -> [_ w163]
                  tunnel: [w160 w161] -> w151
                  frame False {
                  }
                  frame True {
                    n64 = Insert Into Array(array=w166, new element=w165) -> (w162:string[])  [unwired: 1 in]
                    n65 = property class="CmbBox"(reference=w163, error in=w164, "Strings[]"=w162) -> (error out=w161:errorcluster)  [unwired: 1 out]
                  }
                }
              }
              event "Load Excel": Value Change {
                n66 = event-data() -> ()  [unwired: 1 in, 6 out]
              }
              event "ComboBox.SelectTestSequence": Value Change {
                n67 = event-data() -> ("NewVal"=w171:string)  [unwired: 1 in]
                n68 = Unbundle By Name(w179) -> ("Seq.AllList"=w178:T2[])
                n69 = To Lower Case(string=w171) -> (all lower case string=w170:string)
                n70 = case shown="\"all\"" w170 {
                  tunnel: w178 -> [w183 w190]
                  tunnel: w171 -> [w182 _]
                  tunnel: [w181 T2[] []] -> w176
                  tunnel: [w180 w190] -> w173
                  frame Default {
                    n71 = for {
                      tunnel: w183 -> [w186] mode=indexing
                      tunnel: w182 -> [w187]
                      tunnel: [w186] -> w180 mode=indexing if=w184
                      tunnel: [w186] -> w181 mode=indexing if=w185
                      n72 = Unbundle By Name(w186) -> ("Seq.TestSequence"=w188:string)
                      n73 = Equal?(x=w188, y=w187) -> (x = y?=w184:bool)
                      n74 = Not(x=w184) -> (.not. x?=w185:bool)
                    }
                  }
                  frame "all" {
                  }
                }
                n75 = Bundle By Name(cluster=w179, "Seq.ShownList"=w173, "Seq.HiddenList"=w176) -> (w177:T12)
                n76 = property on="MCListbox.Sequence List" class="Arr (strict)"(error in=w175, "Value"=w173) -> (error out=w174:errorcluster)  [unwired: 1 in, 1 out]
              }
              event "MCListbox.Sequence List": Value Change {
                n77 = event-data() -> ("NewVal"=w191:T2[])  [unwired: 1 in, 5 out]
                n78 = Unbundle By Name(w194) -> ("Seq.HiddenList"=w192:T2[])
                n79 = Build Array (concatenate)(w191, w192) -> (w193:T2[])
                n80 = Bundle By Name(cluster=w194, "Seq.AllList"=w193, "Seq.ShownList"=w191) -> (w195:T12)
              }
              event "Save": Value Change {
                n81 = event-data() -> ()  [unwired: 1 in, 6 out]
                n82 = Unbundle By Name(w204) -> ("Seq.AllList"=w203:T2[])
                n83 = for {
                  tunnel: w203 -> [w207] mode=indexing
                  tunnel: w203 -> [w206] mode=indexing
                  tunnel: [w206] -> w200 mode=indexing if=w205
                  n84 = Unbundle By Name(w207) -> ("Seq.Run"=w205:bool)
                }
                n85 = call "eFGV - Sequence Data.vi"("States"=State_-_eFGV."Write", "Error In"=w202, "Sequence Data"=w200) -> ("Error Out"=w201:errorcluster)  [unwired: 6 in, 2 out]
              }
              event "Btn.RunSequence": Value Change {
                n86 = event-data() -> ()  [unwired: 1 in, 1 out]
                n87 = property on="MCListbox.Sequence List" class="Arr (strict)"(error in=w213) -> (error out=w211:errorcluster, "Value"=w212:T2[])  [unwired: 1 in, 1 out]
                n88 = for {
                  tunnel: w212 -> [w217] mode=indexing
                  tunnel: [w216] -> w209 mode=indexing
                  n89 = Bundle By Name(cluster=w217, "Seq.Run"=TRUE) -> (w216:T2)
                }
                n90 = property on="MCListbox.Sequence List" class="Arr (strict)"(error in=w211, "Val(Sgnl)"=w209) -> (error out=w210:errorcluster)  [unwired: 1 in, 1 out]
              }
              event "Btn.ClearRunSequence": Value Change {
                n91 = event-data() -> ()  [unwired: 1 in, 1 out]
                n92 = property on="MCListbox.Sequence List" class="Arr (strict)"(error in=w223) -> (error out=w221:errorcluster, "Value"=w222:T2[])  [unwired: 1 in, 1 out]
                n93 = for {
                  tunnel: w222 -> [w227] mode=indexing
                  tunnel: [w226] -> w219 mode=indexing
                  n94 = Bundle By Name(cluster=w227, "Seq.Run"=FALSE) -> (w226:T2)
                }
                n95 = property on="MCListbox.Sequence List" class="Arr (strict)"(error in=w221, "Val(Sgnl)"=w219) -> (error out=w220:errorcluster)  [unwired: 1 in, 1 out]
              }
              event "Test System": Value Change {
                n96 = event-data() -> ("NewVal"=w233:string, "CtlRef"=w237:refnum<vi>)  [unwired: 1 in]
                n97 = property class="CmbBox"(reference=w237, error in=w236) -> (reference out=w231:refnum<vi>, error out=w232:errorcluster, "Strings[]"=w229:string[])
                n98 = call "Gen - Remove Empty String Array.vi"("Data Array"=w229) -> ("Data Out"=w228:string[])  [unwired: 10 in]
                n99 = call "Search Unsorted 1D Array.vim"("element"=w233, "unsorted 1D array"=w228) -> ("index of element"=w235:i32)  [unwired: 9 in]
                n100 = Less Than 0?(x=w235) -> (x < 0?=w234:bool)
                n101 = case shown="True" w234 {
                  tunnel: w228 -> [_ w246]
                  tunnel: w233 -> [_ w245]
                  tunnel: w232 -> [w240 w244]
                  tunnel: w231 -> [_ w243]
                  tunnel: [w240 w241] -> w230
                  frame False {
                  }
                  frame True {
                    n102 = Insert Into Array(array=w246, new element=w245) -> (w242:string[])  [unwired: 1 in]
                    n103 = property class="CmbBox"(reference=w243, error in=w244, "Strings[]"=w242) -> (error out=w241:errorcluster)  [unwired: 1 out]
                  }
                }
              }
              event "Add SN": Value Change {
                n104 = event-data() -> ()  [unwired: 1 in, 6 out]
                n105 = property on="Input SN" class="Str"(error in=w252) -> (error out=w251:errorcluster, "Value"=w249:string)  [unwired: 1 in, 1 out]
                n106 = Empty String/Path?(string/path=w249) -> (empty?=w250:bool)
                n107 = case shown="False" w250 {
                  tunnel: w251 -> [w256 w270]
                  tunnel: w249 -> [w258 _]
                  tunnel: [w257 w270] -> w248
                  frame False {
                    n108 = property on="List SN" class="LstBox (strict)"(error in=w256) -> (error out=w255:errorcluster, "Item Names"=w254:string[])  [unwired: 1 in, 1 out]
                    n109 = call "Search Unsorted 1D Array.vim"("element"=w258, "unsorted 1D array"=w254) -> ("index of element"=w260:i32)  [unwired: 9 in]
                    n110 = Less Than 0?(x=w260) -> (x < 0?=w259:bool)
                    n111 = case shown="True" w259 {
                      tunnel: w255 -> [w261 w265]
                      tunnel: w254 -> [_ w269]
                      tunnel: w258 -> [_ w268]
                      tunnel: [w261 w266] -> w257
                      frame False {
                        n112 = One Button Dialog(message="Serial Number already exist") -> ()  [unwired: 1 in, 1 out]
                      }
                      frame True {
                        n113 = Insert Into Array(array=w269, new element=w268) -> (w263:string[])  [unwired: 1 in]
                        n114 = property on="List SN" class="LstBox (strict)"(error in=w265, "Item Names"=w263) -> (error out=w264:errorcluster)  [unwired: 1 in, 1 out]
                        n115 = property on="Input SN" class="Str"(error in=w264, "Value"="" ("Input SN")) -> (error out=w266:errorcluster)  [unwired: 1 in, 1 out]
                      }
                    }
                  }
                  frame True {
                    n116 = One Button Dialog(message="Serial number empty") -> ()  [unwired: 1 in, 1 out]
                  }
                }
              }
              event "List SN": Mouse Down {
                n117 = event-data() -> ("CtlRef"=w278:refnum<vi>)  [unwired: 1 in, 7 out]
                n118 = property class="LstBox (strict)"(reference=w278, error in=w279) -> (error out=w275:errorcluster, "FocusRow"=w276:i32, "Item Names"=w277:string[])  [unwired: 1 out]
                n119 = Index Array(array=w277, index=w276) -> (element=w274:string)
                n120 = property on="Input SN" class="Str"(error in=w275, "Value"=w274) -> (error out=w273:errorcluster)  [unwired: 1 in, 1 out]
              }
              event "Remove SN": Value Change {
                n121 = event-data() -> ()  [unwired: 1 in, 6 out]
                n122 = property on="List SN" class="LstBox (strict)"(error in=w289) -> (error out=w288:errorcluster, "Item Names"=w284:string[])  [unwired: 1 in, 1 out]
                n123 = property on="Input SN" class="Str"(error in=w288) -> (error out=w285:errorcluster, "Value"=w287:string)  [unwired: 1 in, 1 out]
                n124 = call "Search Unsorted 1D Array.vim"("element"=w287, "unsorted 1D array"=w284) -> ("index of element"=w283:i32)  [unwired: 9 in]
                n125 = Less Than 0?(x=w283) -> (x < 0?=w286:bool)
                n126 = case shown="False" w286 {
                  tunnel: w285 -> [w294 w299]
                  tunnel: w284 -> [w298 _]
                  tunnel: w283 -> [w297 _]
                  tunnel: [w291 w299] -> w282
                  frame False {
                    n127 = Delete From Array(array=w298, length=1, index=w297) -> (array with subset deleted=w295:string[])  [unwired: 1 out]
                    n128 = property on="List SN" class="LstBox (strict)"(error in=w294, "Item Names"=w295) -> (error out=w293:errorcluster)  [unwired: 1 in, 1 out]
                    n129 = property on="Input SN" class="Str"(error in=w293, "Value"="" ("Input SN")) -> (error out=w291:errorcluster)  [unwired: 1 in, 1 out]
                  }
                  frame True {
                    n130 = One Button Dialog(message="No matching SN to remove") -> ()  [unwired: 1 in, 1 out]
                  }
                }
              }
              event "Rework": Value Change {
                n131 = event-data() -> ("NewVal"=w304:bool)  [unwired: 1 in]
                n132 = case shown="False" w304 {
                  tunnel: [FALSE ("Visible") TRUE ("Visible")] -> w303
                  tunnel: [T17."Disabled" ("Disabled") T17."Enabled" ("Disabled")] -> w302
                  frame False {
                  }
                  frame True {
                  }
                }
                n133 = property on="NCR No." class="Str"(error in=w307, "Visible"=w303, "DisabledEnum"=w302) -> (error out=w306:errorcluster)  [unwired: 1 in, 1 out]
                n134 = property on="Ref Order No." class="DigNum (strict)"(error in=w306, "Visible"=w303, "DisabledEnum"=w302) -> (error out=w305:errorcluster)  [unwired: 1 in, 1 out]
              }
              event "Add Sensor": Value Change {
                n135 = event-data() -> ()  [unwired: 1 in, 5 out]
                n136 = call "Popup - Add Sensor.vi"() -> ("Output Sensor"=w313:T21, "Cancelled?"=w315:bool)  [unwired: 10 in]
                n137 = case shown="False" w315 {
                  tunnel: w316 -> [w333 w334]
                  tunnel: [w329 w334] -> w314
                  tunnel: w313 -> [w328 _]
                  frame False {
                    n138 = Unbundle By Name(w328) -> ("Type"=w320:string, "ID"=w321:string, "Description"=w322:string, "Serial No."=w323:string, "Low Pressure?"=w327:bool)
                    n139 = Select(t="Y", s=w327, f="N") -> (s? t:f=w324:string)
                    n140 = Build Array(w320, w321, w322, w323, w324) -> (w319:string[])
                    n141 = property on="Table.Sensor" class="MCListbox (strict)"(error in=w333) -> (error out=w331:errorcluster, "ItemNames"=w332:string[][])  [unwired: 1 in, 1 out]
                    n142 = Insert Into Array(array=w332, new element=w319) -> (w330:string[][])  [unwired: 2 in]
                    n143 = property on="Table.Sensor" class="MCListbox (strict)"(error in=w331, "ItemNames"=w330) -> (error out=w329:errorcluster)  [unwired: 1 in, 1 out]
                  }
                  frame True {
                  }
                }
              }
              event "Add Tool": Value Change {
                n144 = event-data() -> ()  [unwired: 1 in, 5 out]
                n145 = call "Popup - Tools.vi"() -> ("Output Tools"=w335:T22, "Cancelled?"=w336:bool)  [unwired: 10 in]
                n146 = case shown="False" w336 {
                  tunnel: w338 -> [w351 w352]
                  tunnel: [w347 w352] -> w337
                  tunnel: w335 -> [w346 _]
                  frame False {
                    n147 = Unbundle By Name(w346) -> ("Type"=w342:string, "ID"=w343:string, "Description"=w344:string, "Serial No."=w345:string)
                    n148 = Build Array(w342, w343, w344, w345) -> (w341:string[])
                    n149 = property on="Table.Tool" class="MCListbox (strict)"(error in=w351) -> (error out=w349:errorcluster, "ItemNames"=w350:string[][])  [unwired: 1 in, 1 out]
                    n150 = Insert Into Array(array=w350, new element=w341) -> (w348:string[][])  [unwired: 2 in]
                    n151 = property on="Table.Tool" class="MCListbox (strict)"(error in=w349, "ItemNames"=w348) -> (error out=w347:errorcluster)  [unwired: 1 in, 1 out]
                  }
                  frame True {
                  }
                }
              }
              event "Remove Sensor": Value Change {
                n152 = event-data() -> ()  [unwired: 1 in, 5 out]
                n153 = property on="Table.Sensor" class="MCListbox (strict)"(error in=w360) -> (error out=w359:errorcluster, "FocusRow"=w356:i32)  [unwired: 1 in, 1 out]
                n154 = property on="Table.Sensor" class="MCListbox (strict)"(error in=w359) -> (error out=w354:errorcluster, "ItemNames"=w358:string[][])  [unwired: 1 in, 1 out]
                n155 = Delete From Array(array=w358, length=1, index (row)=w356) -> (array with subset deleted=w355:string[][])  [unwired: 1 in, 1 out]
                n156 = property on="Table.Sensor" class="MCListbox (strict)"(error in=w354, "ItemNames"=w355) -> (error out=w353:errorcluster)  [unwired: 1 in, 1 out]
              }
              event "Remove Tools": Value Change {
                n157 = event-data() -> ()  [unwired: 1 in, 5 out]
                n158 = property on="Table.Tool" class="MCListbox (strict)"(error in=w370) -> (error out=w369:errorcluster, "FocusRow"=w366:i32)  [unwired: 1 in, 1 out]
                n159 = property on="Table.Tool" class="MCListbox (strict)"(error in=w369) -> (error out=w364:errorcluster, "ItemNames"=w368:string[][])  [unwired: 1 in, 1 out]
                n160 = Delete From Array(array=w368, length=1, index (row)=w366) -> (array with subset deleted=w365:string[][])  [unwired: 1 in, 1 out]
                n161 = property on="Table.Tool" class="MCListbox (strict)"(error in=w364, "ItemNames"=w365) -> (error out=w363:errorcluster)  [unwired: 1 in, 1 out]
              }
              event "Remove Additional Ref Procedure": Value Change {
                n162 = event-data() -> ()  [unwired: 1 in, 5 out]
                n163 = property on="Table.Procedure No./Ref." class="MCListbox (strict)"(error in=w380) -> (error out=w379:errorcluster, "FocusRow"=w376:i32)  [unwired: 1 in, 1 out]
                n164 = property on="Table.Procedure No./Ref." class="MCListbox (strict)"(error in=w379) -> (error out=w374:errorcluster, "ItemNames"=w378:string[][])  [unwired: 1 in, 1 out]
                n165 = Delete From Array(array=w378, length=1, index (row)=w376) -> (array with subset deleted=w375:string[][])  [unwired: 1 in, 1 out]
                n166 = property on="Table.Procedure No./Ref." class="MCListbox (strict)"(error in=w374, "ItemNames"=w375) -> (error out=w373:errorcluster)  [unwired: 1 in, 1 out]
              }
              event "Add Additional Ref Procedure": Value Change {
                n167 = event-data() -> ()  [unwired: 1 in, 5 out]
                n168 = local read "Listbox.Additional Procedures No./Ref."() -> (w386:string)
                n169 = local read "Listbox.Rev."() -> (w385:string)
                n170 = local read "Listbox.PSL"() -> (w387:string)
                n171 = Empty String/Path?(string/path=w386) -> (empty?=w393:bool)
                n172 = Empty String/Path?(string/path=w385) -> (empty?=w392:bool)
                n173 = Empty String/Path?(string/path=w387) -> (empty?=w391:bool)
                n174 = Build Array(w386, w385, w387) -> (w384:string[])
                n175 = Compound Arithmetic op=OR(w393, w392, w391) -> (w383:bool)
                n176 = case shown="False" w383 {
                  tunnel: w389 -> [w401 w403]
                  tunnel: [w396 w403] -> w388
                  tunnel: w384 -> [w399 _]
                  frame False {
                    w395 = "" ("Listbox.Additional Procedures No./Ref.")
                    n177 = property on="Table.Procedure No./Ref." class="MCListbox (strict)"(error in=w401) -> (error out=w397:errorcluster, "ItemNames"=w400:string[][])  [unwired: 1 in, 1 out]
                    n178 = local write "Listbox.Additional Procedures No./Ref."(w395) -> ()
                    n179 = Insert Into Array(array=w400, new element=w399) -> (w398:string[][])  [unwired: 2 in]
                    n180 = property on="Table.Procedure No./Ref." class="MCListbox (strict)"(error in=w397, "ItemNames"=w398) -> (error out=w396:errorcluster)  [unwired: 1 in, 1 out]
                    n181 = local write "Listbox.Rev."(w395) -> ()
                    n182 = local write "Listbox.PSL"(w395) -> ()
                  }
                  frame True {
                    n183 = One Button Dialog(message="EMPTY PARAMETER") -> ()  [unwired: 1 in, 1 out]
                  }
                }
              }
              event User Event {
                n184 = event-data() -> ()  [unwired: 1 in, 5 out]
              }
              event "Enum.Max Start Hold Pressure": Value Change {
                n185 = event-data() -> ("NewVal"=w410:enum16{"%", "psi"})  [unwired: 1 in]
                n186 = case shown="\"%\", Default" w410 {
                  tunnel: [100.0 ("Data Entry Limits:Maximum") 30000.0 ("Data Entry Limits:Maximum")] -> w409
                  tunnel: [0.0 ("Data Entry Limits:Minimum") 0.0 ("Data Entry Limits:Minimum")] -> w408
                  frame "%", Default {
                  }
                  frame "psi" {
                  }
                }
                n187 = property on="Max Start Hold Pressure" class="DigNum (strict)"(error in=w412, "Maximum"=w409, "Minimum"=w408) -> (error out=w411:errorcluster)  [unwired: 1 in, 1 out]
              }
              event "Enum.Permitted Hold Pressure Drop": Value Change {
                n188 = event-data() -> ("NewVal"=w421:enum16{"%", "psi"})  [unwired: 1 in]
                n189 = case shown="\"%\", Default" w421 {
                  tunnel: [100.0 ("Data Entry Limits:Maximum") 30000.0 ("Data Entry Limits:Maximum")] -> w420
                  tunnel: [0.0 ("Data Entry Limits:Minimum") 0.0 ("Data Entry Limits:Minimum")] -> w419
                  frame "%", Default {
                  }
                  frame "psi" {
                  }
                }
                n190 = property on="Permitted Hold Pressure Drop" class="DigNum (strict)"(error in=w423, "Maximum"=w420, "Minimum"=w419) -> (error out=w422:errorcluster)  [unwired: 1 in, 1 out]
              }
            }
            n191 = Bundle By Name(cluster=w116, "Event Ref"=w111) -> (w112:T12)
          }
          frame "Get product info" {
            n192 = call "FGV - Data Path.vi"("FGV State"=State_-_FGV."Read", "Error In"=w434) -> ("Error Out"=w436:errorcluster, "Path Out"=w437:path)  [unwired: 8 in]
            n193 = Unbundle By Name(w432) -> ("Product Category"=w431:string)
            n194 = Build Path(base path=w437, name or relative path="Data\\Procedure") -> (appended path=w440:path)
            n195 = Build Path(base path=w440, name or relative path="Product Category.ini") -> (appended path=w438:path)
            n196 = call <vilib>:"Open Config Data.vi"("error in (no error)"=w436, "configuration file path"=w438) -> ("error out"=w453:errorcluster, "refnum"=w452:T20)  [unwired: 7 in, 1 out]
            n197 = for {
              tunnel: w453 -> [w460]
              tunnel: w452 -> [w459]
              tunnel: w431 -> [w458]
              tunnel: string[] ["Procedure No", "Rev", "PSL", "Working Pressure"] -> [w457] mode=indexing
              tunnel: [w456] -> w446 mode=indexing
              tunnel: [w455] -> w450
              tunnel: [w454] -> w449
              n198 = call-poly <vilib>:"Read Key.vi"("section"=w458, "error in (no error)"=w460, "key"=w457, "refnum"=w459) -> ("error out"=w455:errorcluster, "value"=w456:string, "refnum out"=w454:T20)  [unwired: 4 in, 1 out]
            }
            n199 = Index Array(array=w446) -> (element #2=w445:string, element #3=w444:string, element #4=w443:string)  [unwired: 4 in, 1 out]
            n200 = call <vilib>:"Close Config Data.vi"("error in (no error)"=w450, "refnum"=w449) -> ("error out"=w435:errorcluster)  [unwired: 8 in, 1 out]
            n201 = property on="Rev." class="Str"(error in=w435, "Value"=w445) -> (error out=w448:errorcluster)  [unwired: 1 in, 1 out]
            n202 = property on="PSL" class="Str"(error in=w448, "Value"=w444) -> (error out=w447:errorcluster)  [unwired: 1 in, 1 out]
            n203 = property on="Working Pressure" class="Str"(error in=w447, "Value"=w443) -> (error out=w433:errorcluster)  [unwired: 1 in, 1 out]
          }
          frame "Read sequence csv" {
            n204 = disable-structure shown="Enabled" {
              disable-tunnel: [w472 w479] -> w462
              disable-tunnel: w461 -> [w471 w479]
              frame Disabled {
                (unwired) path "C:/Users/SNG_THINKPAD/Documents/g159-one-subsea-test-pressure-monitoring-system/VI/HMI/Data/Data/Procedure" ("configuration file path")
                n205 = call "FGV - Data Path.vi"("FGV State"=State_-_FGV."Read", "Error In"=w471) -> ("Error Out"=w466:errorcluster, "Path Out"=w469:path)  [unwired: 8 in]
                n206 = Build Path(base path=w469, name or relative path="Data\\Procedure") -> (appended path=w467:path)
                n207 = Concatenate Strings(".csv" ("string")) -> (w477:string)  [unwired: 1 in]
                n208 = Build Path(base path=w467, name or relative path=w477) -> (appended path=w478:path)
                n209 = call-poly <vilib>:"Read Delimited Spreadsheet.vi"("file path (dialog if empty)"=w478, "error in (no error)"=w466) -> ("all rows"=w475:string[][], "error out"=w473:errorcluster)  [unwired: 8 in, 4 out]
                n210 = call "Get sequence list.vi"("all rows"=w475) -> ("Output sequence"=w474:T2[])
              }
              frame Enabled {
              }
            }
          }
          frame "Get Sequence List" {
            n211 = property on="Procedure No./Ref." class="CmbBox"() -> ("Value"=w483:string)  [unwired: 2 in, 2 out]
            n212 = Unbundle By Name(w485) -> ("File String"=w484:string[])
            n213 = for {
              tunnel: w484 -> [w492] mode=indexing
              tunnel: w483 -> [w493]
              tunnel: [w492] -> w482
              tunnel: [w490] -> w480
              stop <- w490 continue-if-true
              n214 = Match Pattern(string=w492, regular expression=w493) -> (match substring=w491:string)  [unwired: 1 in, 3 out]
              n215 = Empty String/Path?(string/path=w491) -> (empty?=w490:bool)
            }
            n216 = String To Path(string=w482) -> (path=w481:path)
            n217 = case shown="False" w480 {
              tunnel: w489 -> [w512 w514]
              tunnel: [w501 w514] -> w488
              tunnel: w481 -> [w494 _]
              tunnel: w485 -> [w496 w513]
              tunnel: [w496 w513] -> w487
              frame False {
                n218 = call <vilib>:"Create Report.vi"("window state (normal)"=T18."no change", "report type"=Report_Type."Excel", "template (empty)"=w494, "error in (no error)"=w512) -> ("report out"=w508:refnum<class "NI_report.lvclass">, "error out"=w509:errorcluster)  [unwired: 10 in]
                n219 = call <vilib>:"Excel Get Worksheet.vi"("report in"=w508, "worksheet index (0)"=0, "error in (no error)"=w509) -> ("report out"=w505:refnum<class "NI_report.lvclass">, "error out"=w506:errorcluster)  [unwired: 11 in]
                n220 = call-poly <vilib>:"Excel Get Data.vi"("report in"=w505, "data type"=string[][] [], "error in (no error)"=w506) -> ("report out"=w502:refnum<class "NI_report.lvclass">, "data"=w495:string[][], "error out"=w503:errorcluster)  [unwired: 10 in]
                n221 = call "Sequence Data 2d Array to Cluster.vi"("data"=w495) -> ("Array"=w497:T2[])
                n222 = call-dynamic "Dispose Report.vi"("report in"=w502, "error in (no error)"=w503) -> ("error out"=w500:errorcluster)  [unwired: 13 in]
                n223 = call "Gen - Get Unique Value.vi"("data"=w495) -> ("Unique Values"=w498:string[])
                n224 = property on="ComboBox.SelectTestSequence" class="CmbBox"(error in=w500, "Strings[]"=w498) -> (error out=w499:errorcluster)  [unwired: 1 in, 1 out]
                n225 = property on="MCListbox.Sequence List" class="Arr (strict)"(error in=w499, "Val(Sgnl)"=w497) -> (error out=w501:errorcluster)  [unwired: 1 in, 1 out]
              }
              frame True {
              }
            }
          }
          frame "Get Transaction Info" {
            n226 = local read "Customer Description"() -> (w520:string)
            n227 = local read "Transaction Number"() -> (w516:u32)
            n228 = local read "Material Description"() -> (w524:string)
            n229 = local read "Order Number"() -> (w517:u32)
            n230 = local read "Ref Order No."() -> (w527:dbl)
            n231 = local read "Sales Order"() -> (w522:u32)
            n232 = local read "Customer"() -> (w519:u32)
            n233 = local read "BOM Rev."() -> (w529:dbl)
            n234 = local read "Quantity"() -> (w518:u16)
            n235 = local read "NCR No."() -> (w526:string)
            n236 = local read "Item No."() -> (w528:u32)
            n237 = local read "Material"() -> (w523:u32)
            n238 = local read "Rework"() -> (w525:bool)
            n239 = local read "Project"() -> (w521:string)
            n240 = Bundle("Transaction Number"=w516, "Order Number"=w517, "Quantity"=w518, "Customer"=w519, "Customer Description"=w520, "Project"=w521, "Sales Order"=w522, "Material"=w523, "Material Description"=w524, "Rework"=w525, "NCR No."=w526, "Ref Order No."=w527, "Item No."=w528, "BOM Rev."=w529) -> (w515:T23)  [unwired: 1 in]
            n241 = Bundle By Name(cluster=w532, "Data to Execute.Transaction Info"=w515) -> (w530:T12)
          }
          frame "Get product Info" {
            n242 = local read "Test System Description"() -> (w541:string)
            n243 = local read "Procedure No./Ref."() -> (w539:string)
            n244 = local read "Product Category"() -> (w538:string)
            n245 = local read "Working Pressure"() -> (w542:string)
            n246 = local read "Pressure Unit"() -> (w543:string)
            n247 = local read "Test System"() -> (w540:string)
            n248 = local read "Rev."() -> (w544:string)
            n249 = local read "PSL"() -> (w545:string)
            n250 = Bundle("Product Category"=w538, "Procedure No./Ref."=w539, "Test System"=w540, "Test System Description"=w541, "Working Pressure"=w542, "Pressure Unit"=w543, "Rev."=w544, "PSL"=w545) -> (w536:T24)  [unwired: 1 in]
            n251 = Bundle By Name(cluster=w546, "Data to Execute.Product Info"=w536) -> (w537:T12)
          }
          frame "Get Misc - Additional Refs" {
            n252 = property on="Table.Procedure No./Ref." class="MCListbox (strict)"(error in=w552) -> (error out=w551:errorcluster, "ItemNames"=w549:string[][])  [unwired: 1 in, 1 out]
            n253 = Bundle By Name(cluster=w553, "Data to Execute.Misc - Additional Refs"=w549) -> (w550:T12)
          }
          frame "Get Misc - Sensors" {
            n254 = property on="Table.Sensor" class="MCListbox (strict)"(error in=w558) -> (error out=w557:errorcluster, "ItemNames"=w555:string[][])  [unwired: 1 in, 1 out]
            n255 = Bundle By Name(cluster=w559, "Data to Execute.Misc - Sensors"=w555) -> (w556:T12)
          }
          frame "Get Misc - Tools" {
            n256 = property on="Table.Tool" class="MCListbox (strict)"(error in=w564) -> (error out=w563:errorcluster, "ItemNames"=w561:string[][])  [unwired: 1 in, 1 out]
            n257 = Bundle By Name(cluster=w565, "Data to Execute.Misc - Tools"=w561) -> (w562:T12)
          }
          frame "Get Misc - Accept Criteria" {
            n258 = local read "Enum.Permitted Hold Pressure Drop"() -> (w572:enum16{"%", "psi"})
            n259 = local read "Enum.Max Start Hold Pressure"() -> (w570:enum16{"%", "psi"})
            n260 = local read "Permitted Hold Pressure Drop"() -> (w571:dbl)
            n261 = local read "Max Start Hold Pressure"() -> (w569:dbl)
            n262 = Bundle("Max Start Hold Pressure"=w569, "Enum.Max Start Hold Pressure"=w570, "Permitted Hold Pressure Drop"=w571, "Enum.Permitted Hold Pressure Drop"=w572) -> (w567:T25)  [unwired: 1 in]
            n263 = Bundle By Name(cluster=w573, "Data to Execute.Acceptance Criteria Info"=w567) -> (w568:T12)
          }
          frame "Get Misc - Execution" {
            n264 = local read "Auto Set Marker"() -> (w579:bool)
            n265 = local read "Auto Stop Test"() -> (w578:bool)
            n266 = Bundle("Auto Set Marker"=w579, "Auto Stop Test"=w578) -> (w576:T26)  [unwired: 1 in]
            n267 = Bundle By Name(cluster=w580, "Data to Execute.Execution Info"=w576) -> (w577:T12)
          }
          frame "Get Misc - Results" {
            n268 = local read "Output Set Description"() -> (w585:string)
            n269 = local read "ListBox.Output Set"() -> (w586:string)
            n270 = Bundle("ListBox.Output Set"=w586, "Output Set Description"=w585) -> (w583:T27)  [unwired: 1 in]
            n271 = Bundle By Name(cluster=w587, "Data to Execute.Results Info"=w583) -> (w584:T12)
          }
          frame "Get Misc - Notes" {
            n272 = local read "Notes"() -> (w590:string)
            n273 = Bundle By Name(cluster=w592, "Data to Execute.Notes"=w590) -> (w591:T12)
          }
          frame "Check Folder Exist" {
            n274 = call "FGV - Data Path.vi"("FGV State"=State_-_FGV."Read", "Error In"=w608) -> ("Error Out"=w603:errorcluster, "Path Out"=w607:path)  [unwired: 8 in]
            n275 = Unbundle By Name(w605) -> ("Data to Execute.Transaction Info.Transaction Number"=w604:u32)
            n276 = Build Path(base path=w607, name or relative path=path "Results") -> (appended path=w602:path)
            n277 = Number To Decimal String(number=w604) -> (decimal integer string=w601:string)  [unwired: 1 in]
            n278 = Build Path(base path=w602, name or relative path=w601) -> (appended path=w600:path)
            n279 = call <vilib>:"Check if File or Folder Exists.vi"("error in (no error)"=w603, "path"=w600) -> ("error out"=w599:errorcluster, "file or folder exists?"=w598:bool, "dup path"=w595:path)  [unwired: 7 in]
            n280 = case shown="False" w598 {
              tunnel: w599 -> [w611 w614]
              tunnel: [Setup_-_State."Send to Execute" Setup_-_State."Idle"] -> w597
              tunnel: [w609 w613] -> w596
              tunnel: w595 -> [w610 _]
              frame False {
                n281 = Create Folder(path (use dialog)=w610, error in=w611) -> (error out=w609:errorcluster)  [unwired: 1 in, 2 out]
              }
              frame True {
                n282 = call "Gen - Popup Single Button (Auto Close).vi"("Error in"=w614, "Message in"="Transaction number is already used", "Header"="FILE EXISTS") -> ("Error out"=w613:errorcluster)  [unwired: 7 in, 1 out]
              }
            }
          }
          frame "Send to Execute" {
            n283 = Unbundle By Name(w620) -> ("Data to Execute"=w619:T6)
            n284 = call "eFGV - Data to Execute.vi"("Action"=State_-_eFGV."Write", "Error In"=w623, "Data to Execute"=w619) -> ("Error Out"=w622:errorcluster)  [unwired: 7 in, 1 out]
          }
          frame "Close" {
            n285 = Unbundle By Name(w625) -> ("Event Ref"=w624:refnum<event-registration>)
            n286 = Unregister For Events(event registration refnum=w624, error in=w629) -> (error out=w628:errorcluster)
          }
        }
      }
      frame Error {
        n287 = call <vilib>:"Clear Errors.vi"("error in (no error)"=w633) -> ("error out"=w636:errorcluster)  [unwired: 5 in, 1 out]
        n288 = call "Gen - Get Application Kind.vi"("Error In"=w636) -> ("Error Out"=w632:errorcluster, "Application:Kind"=w635:T28)  [unwired: 9 in]
        n289 = Format Into String(error in=w632, w630) -> (resulting string=w631:string)  [unwired: 2 in, 1 out]
        n290 = case shown="\"Development System\"" w635 {
          tunnel: [w640 w645 w649] -> w634
          tunnel: w633 -> [w640 w642 w647]
          tunnel: w631 -> [_ w641 _]
          frame "invalid app kind", Default {
          }
          frame "Run Time System" {
            n291 = control-ref of="This VI"() -> (w643:refnum<vi>)
            n292 = call "eFGV - Generated Error.vi"("eFGV States"=State_-_eFGV."Write", "Error In"=w642, "State"=w641, "This VI"=w643) -> ("Error Out"=w645:errorcluster)  [unwired: 6 in, 1 out]
          }
          frame "Development System" {
            n293 = call <vilib>:"Simple Error Handler.vi"("error in (no error)"=w647) -> ("error?"=w646:bool, "error out"=w648:errorcluster)  [unwired: 4 in, 3 out]
            n294 = case shown="False" w646 {
              tunnel: [w650 w652] -> w649
              tunnel: w648 -> [w650 w651]
              frame False {
              }
              frame True {
                n295 = call <vilib>:"Clear Errors.vi"("error in (no error)"=w651) -> ("error out"=w652:errorcluster)  [unwired: 5 in, 1 out]
              }
            }
          }
        }
      }
    }
    n296 = Wait (ms)(milliseconds to wait=u32 1) -> ()  [unwired: 1 out]
  }
  n297 = while {
    stop <- FALSE stop-if-true
    # "#HIDDEN"
  }
